vi "Facade.vi"(0 "Data In":T6, 2 "Display State In":T3, 3 "Container State":T5) -> (6 "Data Out":T6, 7 "Display State Out":T3, 8 "Action":T2)   [LabVIEW 2017, in "3D Comet.xctl"]
uses:
  <vilib>/Math Plots/3D Math Plots/3D Comet/3D Comet XCtrl/3D Comet.xctl
  <vilib>/Math Plots/3D Math Plots/3D Comet/3D Comet XCtrl/Data.ctl
  <vilib>/Math Plots/3D Math Plots/3D Plot/3D Plot Datatype/3D Plot Datatype.lvclass
  <vilib>/_xctls/Container State.ctl
  <vilib>/Math Plots/3D Math Plots/3D Comet/3D Comet XCtrl/State.ctl
  <vilib>/Math Plots/3D Math Plots/3D Comet/3D Comet/3D Comet.lvclass
  e:/builds/penguin/labview/branches/2017/dev/dist/vi.lib/Math Plots/3D Math Plots/3D Plot/3D Plot/3D Plot.lvclass
  <vilib>/Math Plots/3D Math Plots/3D Plot/Action String/3DMathPlot Ctrl Act Queue.ctl
  <vilib>/Math Plots/3D Math Plots/3D Plot/Action String/3DMathPlot Ctrl Act Cluster.ctl
  <vilib>/Math Plots/3D Math Plots/3D Plot/Action String/3DMathPlot State Class.ctl
  <vilib>/_xctls/Action.ctl
  <vilib>/Math Plots/3D Math Plots/3D Plot/3D Plot/Typedef/Plot Action.ctl
  <vilib>/Math Plots/3D Math Plots/3D Plot/Action String/3DMathPlot Action String.ctl
  <vilib>/_xctls/XControlSupport.lvlib
  <vilib>/Math Plots/3D Math Plots/3D Plot/3D Plot/3D Plot.lvclass
panel:
  out "Export Image":picture
  out "3D Picture Control":refnum<vi>(3d-picture)
  in  "XY Graph":cluster{dbl, dbl}[](graph)
  out "Render Window":refnum<vi>
  in  "Projection Palette":T1
  out "Intensity Graph":dbl[][](graph)
  in  "Color Ramp Palette":cluster{"Active Plot":i32} {"Active Plot" items=["Plot-1"]}
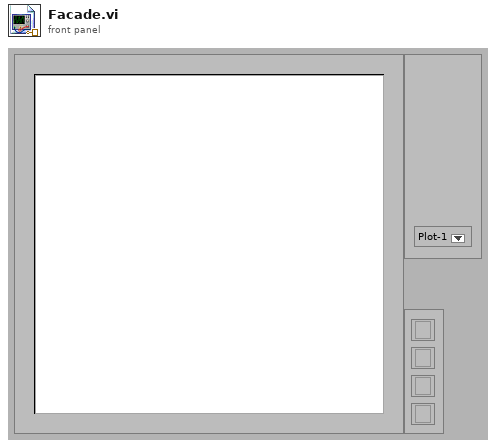
[diagram p1: front panel]
types:
  T1 = cluster{"XY Projection":bool, "XZ Projection":bool, "YZ Projection":bool, "3D Projection":bool}
  T2 = typedef "XControlSupport.lvlib/Action.ctl" = cluster{"Data Changed?":bool, "State Changed?":bool, "Action Name":string}
  T3 = typedef "3D Comet.xctl/State.ctl" = cluster{"3D Comet.lvclass":refnum<class "3D Comet.lvclass">, "Control Ref Queue":T4, "Main Frame Color":u32, "Ramp Palette Color":u32, "Projection Palette Color":u32}
  T4 = typedef "3DMathPlot Ctrl Act Queue.ctl" = refnum<queue>
  T5 = typedef "XControlSupport.lvlib/Container State.ctl" = cluster{"Indicator?":bool, "Run Mode?":bool, " Refnum":refnum<vi>}
  T6 = typedef "3D Comet.xctl/Data.ctl" = refnum<class "3D Plot Datatype.lvclass">[]
  T7 = typedef "3DMathPlot Ctrl Act Cluster.ctl" = cluster{"3D Picture Control":refnum<vi>, "Render Window Refnum":refnum<vi>, "XY Graph":refnum<vi>, "Intensity Graph":refnum<vi>, "Color Legend Palette":refnum<vi>, "Projection Palette":refnum<vi>, "XControl  Ref":refnum<vi>, "Facade Ref":refnum<vi>, "Export Image Ref":refnum<vi>, "Clear Data Flag":bool, "Display State Change Class":T8}
  T8 = typedef "3DMathPlot State Class.ctl" = enum16{"Update All Objects (Undo)", "Update Light Object Only", "Update Axis Object Only", "Update Plot Object Only", "Update Cursor Object Only", "Update Axis Plot Cursor Objects", "No Update"}
  T9 = typedef "3D Plot.lvclass/Plot Action.ctl" = cluster{"Light Action":enum16{"Update", "Remove", "Nothing"}, "Axis Action":enum16{"Update", "Remove", "Nothing"}, "Plot Action":enum16{"Update", "Remove", "Nothing"}, "Cursor Action":enum16{"Update", "Remove", "Nothing"}, "Fast Draw Action":enum16{"Update", "Remove", "Nothing"}}
  T10 = enum32{"Towards X-Y Plane", "Towards X-Z Plane", "Towards Y-Z Plane", "User Defined"}
  T11 = typedef "3D Plot.lvclass/Actual Transform.ctl" = cluster{"Scale Cluster":cluster{"X Scale":sgl, "Y Scale":sgl, "Z Scale":sgl}, "Translate Cluster":cluster{"X Translate":sgl, "Y Translate":sgl, "Z Translate":sgl}, "Actual Range":T12}
  T12 = typedef "3D Plot.lvclass/Range Clusters.ctl" = cluster{"X Range":cluster{"Max X":sgl, "Min X":sgl}, "Y Range":cluster{"Max Y":sgl, "Min Y":sgl}, "Z Range":cluster{"Max Z":sgl, "Min Z":sgl}}
  T13 = typedef "3D Plot.lvclass/Multiplot Representation.ctl" = cluster{"Plot Represention Array":T14[], "Max Range":T12}
  T14 = typedef "3D Plot.lvclass/Plot Representation.ctl" = cluster{"Plot ID":i32, "Plot Range":T12, "Mesh Data":T15, "Dimension":cluster{"X Dimension":i32, "Y Dimension":i32}, "Ramp Range":T12}
  T15 = typedef "3D Plot.lvclass/Mesh Data.ctl" = cluster{"Index Array":u32[], "Vertex Array":cluster{"X":sgl, "Y":sgl, "Z":sgl}[], "Normal Array":cluster{"X":sgl, "Y":sgl, "Z":sgl}[], "Color Index Array":i32[]}
  T16 = typedef "3D Plot.lvclass/Object Cluster.ctl" = cluster{"Root Scene Object":refnum<vi>, "Fast Root Scene Object":refnum<vi>}
  T17 = typedef "3DMathPlot Action String.ctl" = u16
  T18 = typedef "3D Plot.lvclass/Property Cluster.ctl" = cluster{"Graph Property":T19, "Light Property":T23, "Axis Property":T25, "Value Pair Property":T31, "Format Property":T33, "Cursor Property Array":T34, "Appearance Property":T43}
  T19 = typedef "3D Plot.lvclass/Graph Property.ctl" = cluster{"General Property":T20, "View Property":T21, "Grid Plane":T22}
  T20 = typedef "3D Plot.lvclass/General Property.ctl" = cluster{"Plot Area Color":u32, "Fast Draw?":bool, "Clip Data?":bool}
  T21 = typedef "3D Plot.lvclass/View Property.ctl" = cluster{"Projection Mode":enum16{"Orthographic", "Perspective"}, "View Direction":enum32{"Towards X-Y Plane", "Towards X-Z Plane", "Towards Y-Z Plane", "User Defined"}, "User Defined View Direction":cluster{"View Latitude":sgl, "View Longitude":sgl, "View Distance":sgl}}
  T22 = typedef "3D Plot.lvclass/Grid Plane.ctl" = cluster{"Grid Plane Visible":cluster{"Draw Grid Plane X-Y":bool, "Draw Grid Plane Y-Z":bool, "Draw Grid Plane X-Z":bool}, "Grid Antialiasing":bool, "Grid Frame Color":u32}
  T23 = typedef "3D Plot.lvclass/Light Property.ctl" = cluster{"Enable Lighting?":bool, "Ambient Color":u32, "Light Array":T24[]}
  T24 = typedef "3D Plot.lvclass/Light Specific.ctl" = cluster{"Enable Light?":bool, "Light Color":u32, "Light Latitude":sgl, "Light Longitude":sgl, "Light Distance":sgl, "Attenuation":enum16{"None", "Linear", "Quadratic"}}
  T25 = typedef "3D Plot.lvclass/Axis Property.ctl" = cluster{"Caption Property":T26, "Label Property":T27, "Range Property":T28, "Grid Property":T29, "Ticks Property":T30}
  T26 = typedef "3D Plot.lvclass/Caption Property.ctl" = cluster{"Show Caption":cluster{"Show Normal X Caption":bool, "Show Normal Y Caption":bool, "Show Normal Z Caption":bool, "Show Opposite X Caption":bool, "Show Opposite Y Caption":bool, "Show Opposite Z Caption":bool}, "Caption Color":cluster{"Caption Color X":u32, "Caption Color Y":u32, "Caption Color Z":u32}, "Caption Size":cluster{"Caption Size X":u16, "Caption Size Y":u16, "Caption Size Z":u16}, "Caption String":cluster{"Caption X":string, "Caption Y":string, "Caption Z ":string}}
  T27 = typedef "3D Plot.lvclass/Label Property.ctl" = cluster{"Show Label":cluster{"Show Normal X Label":bool, "Show Normal Y Label":bool, "Show Normal Z Label":bool, "Show Opposite X Label":bool, "Show Opposite Y Label":bool, "Show Opposite Z Label":bool}, "Label Color":cluster{"Label Color X":u32, "Label Color Y":u32, "Label Color Z":u32}, "Label Size":cluster{"Label Size X":u16, "Label Size Y":u16, "Labe Size Z":u16}}
  T28 = typedef "3D Plot.lvclass/Range Property.ctl" = cluster{"Range Cluster":T12, "Auto Range":cluster{"Auto Range X":bool, "Auto Range Y":bool, "Auto Range Z":bool}, "Inverted":cluster{"Inverted X":bool, "Inverted Y":bool, "Inverted Z":bool}, "Logarithm":cluster{"Logarithm X":bool, "Logarithm Y":bool, "Logarithm Z":bool}}
  T29 = typedef "3D Plot.lvclass/Grid Property.ctl" = cluster{"Major Grid Visible":cluster{"Draw Major Grid X":bool, "Draw Major Grid Y":bool, "Draw Major Grid Z":bool}, "Major Grid Color":cluster{"Major Grid Color X":u32, "Major Grid Color Y":u32, "Major Grid Color Z":u32}, "Minor Grid Visible":cluster{"Draw Minor Grid X":bool, "Draw Minor Grid Y":bool, "Draw Minor Grid Z":bool}, "Minor Grid Color":cluster{"Minor Grid Color X":u32, "Minor Grid Color Y":u32, "Minor Grid Color Z":u32}}
  T30 = typedef "3D Plot.lvclass/Tick Property.ctl" = cluster{"Major Tick Visible":cluster{"Draw Major Tick X":bool, "Draw Major Tick Y":bool, "Draw Major Tick Z":bool}, "Major Tick Color":cluster{"Major Tick Color X":u32, "Major Tick Color Y":u32, "Major Tick Color Z":u32}, "Major Count":cluster{"Major Count X":u16, "Major Count Y":u16, "Major Count Z":u16}, "Minor Tick Visible":cluster{"Draw Minor Tick X":bool, "Draw Minor Tick Y":bool, "Draw Minor Tick Z":bool}, "Minor Tick Color":cluster{"Minor Tick Color X":u32, "Minor Tick Color Y":u32, "Minor Tick Color Z":u32}, "Minor Count":cluster{"Minor Count X":u16, "Minor Count Y":u16, "Minor Count Z":u16}}
  T31 = typedef "3D Plot.lvclass/Value Pair Property.ctl" = T32[]
  T32 = typedef "3D Plot.lvclass/Value Pair Cluster.ctl" = cluster{"Value Pair Array":cluster{"Value":sgl, "Name":string}[], "Show Tick":bool, "Show Grid":bool, " Label Mode":enum16{"Name", "Value", "None"}}
  T33 = typedef "3D Plot.lvclass/Format Property.ctl" = string[]
  T34 = typedef "3D Plot.lvclass/Cursor Property Array.ctl" = T35[]
  T35 = typedef "3D Plot.lvclass/Cursor Property.ctl" = cluster{"Cursor Visible":bool, "Cursor Enable":bool, "Cursor Position":T36, "Cursor Point":T37, "Cursor Line":T39, "Cursor Plane":T41, "Cursor Text":T42}
  T36 = typedef "3D Plot.lvclass/Cursor Position.ctl" = cluster{"Cursor Plot ID":i32, "Cursor X":sgl, "Cursor Y":sgl, "Cursor Z":sgl, "Cursor Snap To":enum16{"Fixed", "Nearest Plot", "Snap to Plot"}}
  T37 = typedef "3D Plot.lvclass/Cursor Point.ctl" = cluster{"Cursor Point Color":u32, "Cursor Point Size":sgl, "Cursor Point Style":T38}
  T38 = typedef "3D Plot.lvclass/Sprite Type.ctl" = enum16{"None", "Empty Square", "Solid Square", "Empty Diamond", "Solid Diamond", "Empty Circle", "Solid Circle", "Asterisk", "Bold X", "Wireframe Sphere", "Solid Sphere", "Wireframe Cube", "Solid Cube"}
  T39 = typedef "3D Plot.lvclass/Cursor Line.ctl" = cluster{"Cursor Line Color":u32, "Cursor Line Width":sgl, "Cursor Line Style":T40}
  T40 = typedef "3D Plot.lvclass/Line Type.ctl" = enum16{"None", "Solid", "Dash", "Dot", "Dash Dot"}
  T41 = typedef "3D Plot.lvclass/Cursor Plane.ctl" = cluster{"Cursor Plane Color":u32, "Cursor Plane Opacity":sgl, "Draw Cursor Plane X-Z":bool, "Draw Cursor Plane Y-Z":bool, "Draw Cursor Plane X-Y":bool}
  T42 = typedef "3D Plot.lvclass/Cursor Text.ctl" = cluster{"Cursor Text":string, "Cursor Text Size":u16, "Cursor Show Position":bool, "Cursor Show Name":bool, "Cursor Text Color":u32, "Background Color":u32, "Background Opacity":sgl}
  T43 = typedef "3D Plot.lvclass/Apearance Property.ctl" = cluster{"Visibility":T44, "Active Index":cluster{"Active Plot":i32, "Active Cursor":i32, "Active Axis":enum16{"X-axis", "Y-axis", "Z-axis"}, "Active Value Pair":enum16{"X-axis", "Y-axis", "Z-axis"}, "Active Light":enum16{"Light 0", "Light 1", "Light 2", "Light 3"}}, "Backup Data":cluster{"Plot Name":string[]}}
  T44 = typedef "3D Plot.lvclass/Item Visibility.ctl" = cluster{"Projection Palette":bool, "Color Ramp Palette":bool}
  T45 = typedef "LVPoint32TypeDef.ctl" = cluster{"Horizontal":i32, "Vertical":i32}
  T46 = typedef "LVRangeTypeDef.ctl" = cluster{"Minimum":dbl, "Maximum":dbl, "Increment":dbl, "Minor Increment":dbl, "Start":dbl}
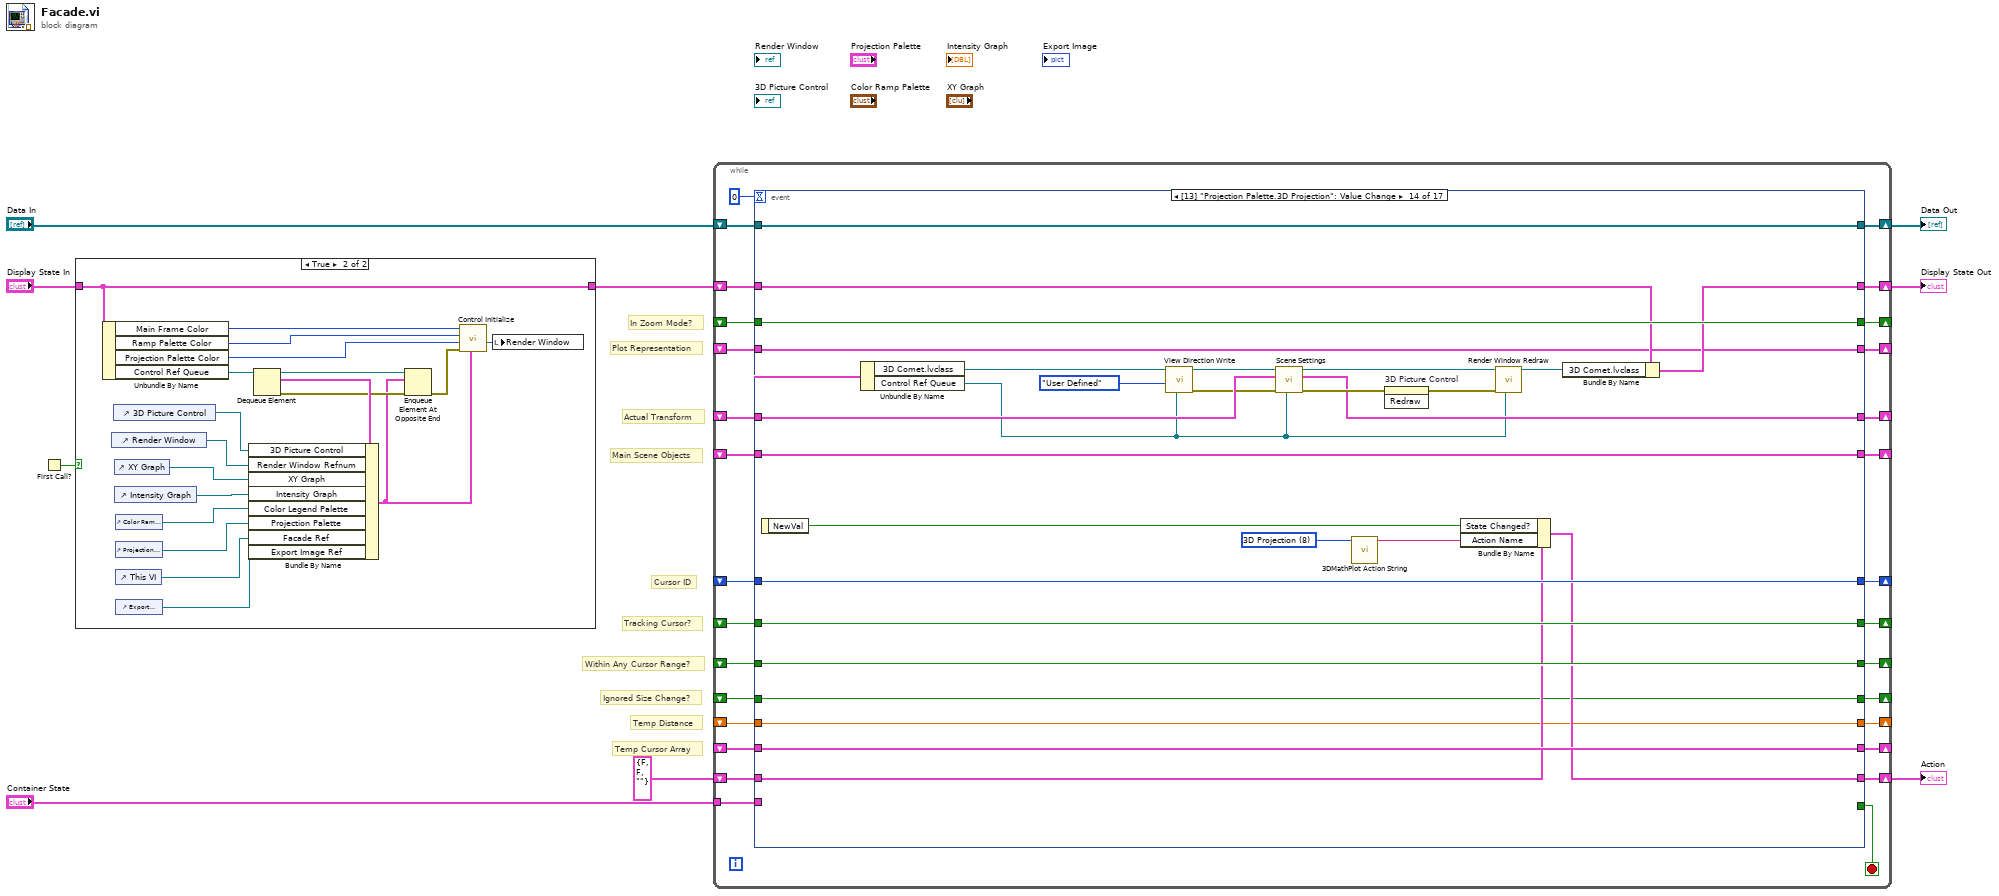
[diagram p0: block diagram]
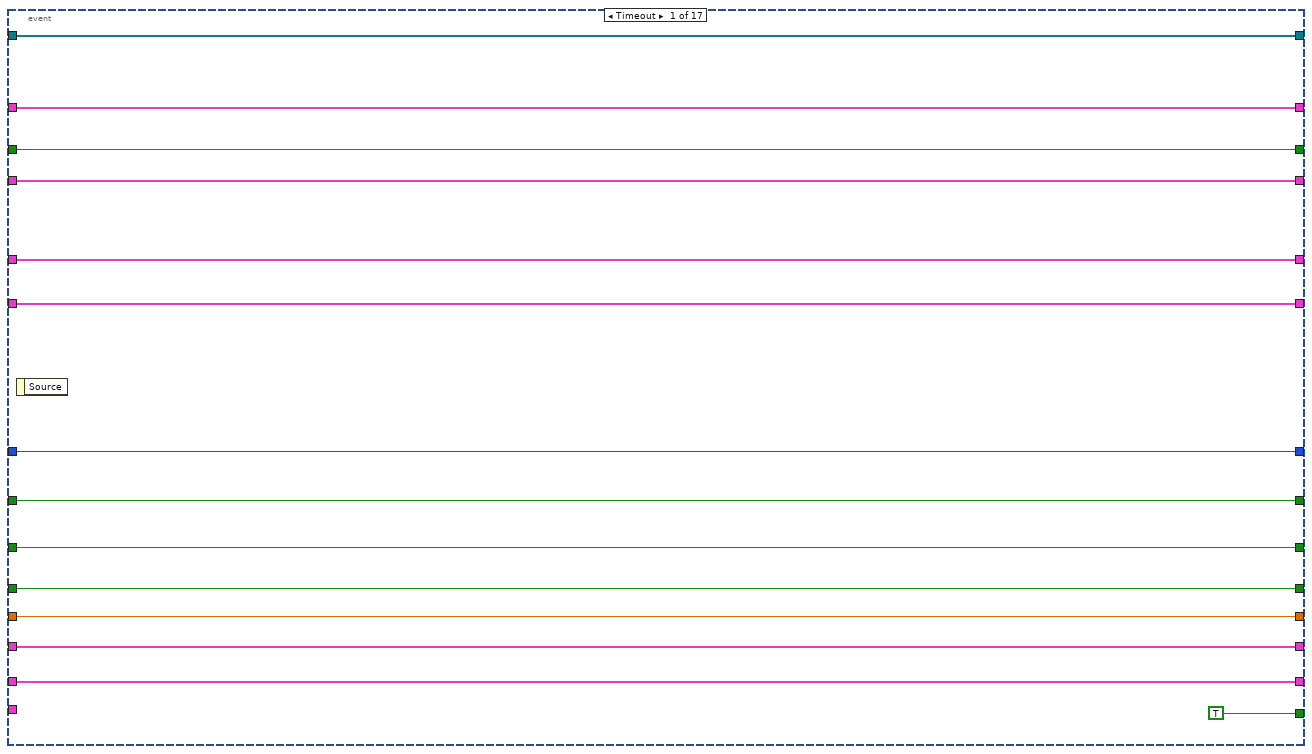
[diagram p3: hidden frame]
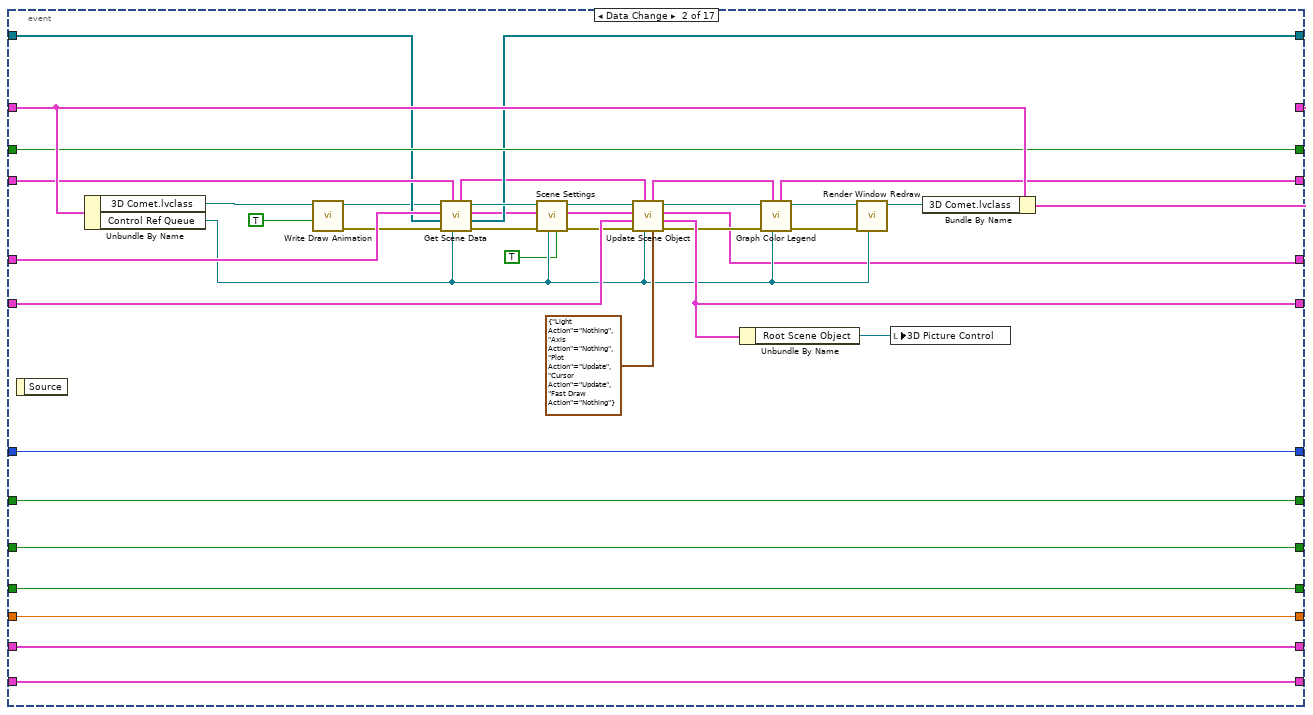
[diagram p4: hidden frame]
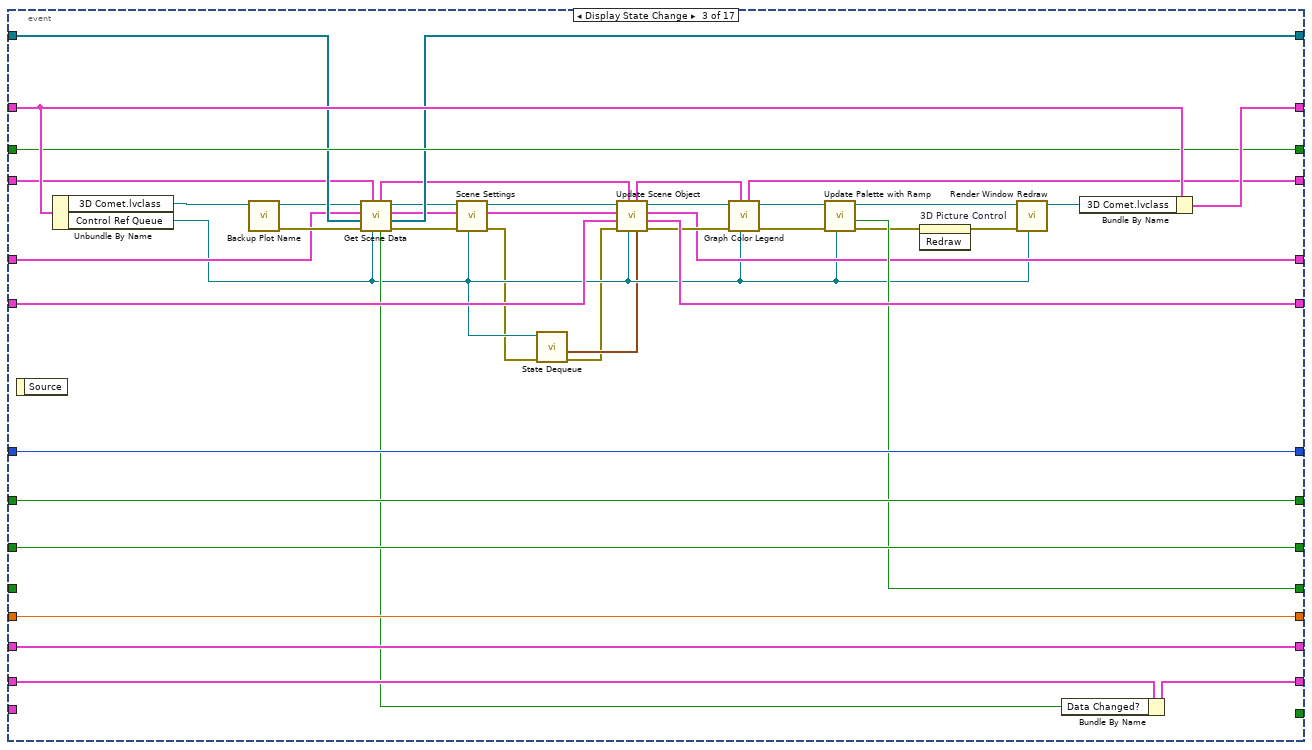
[diagram p5: hidden frame]
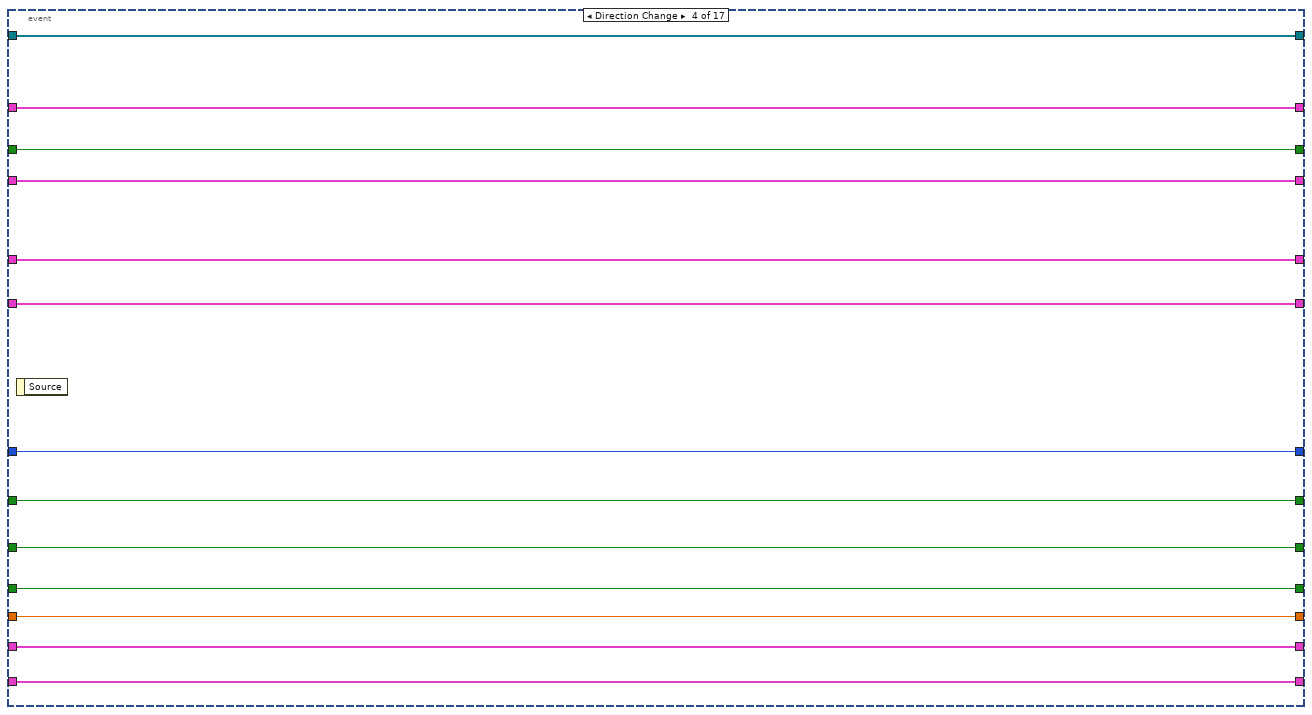
[diagram p6: hidden frame]
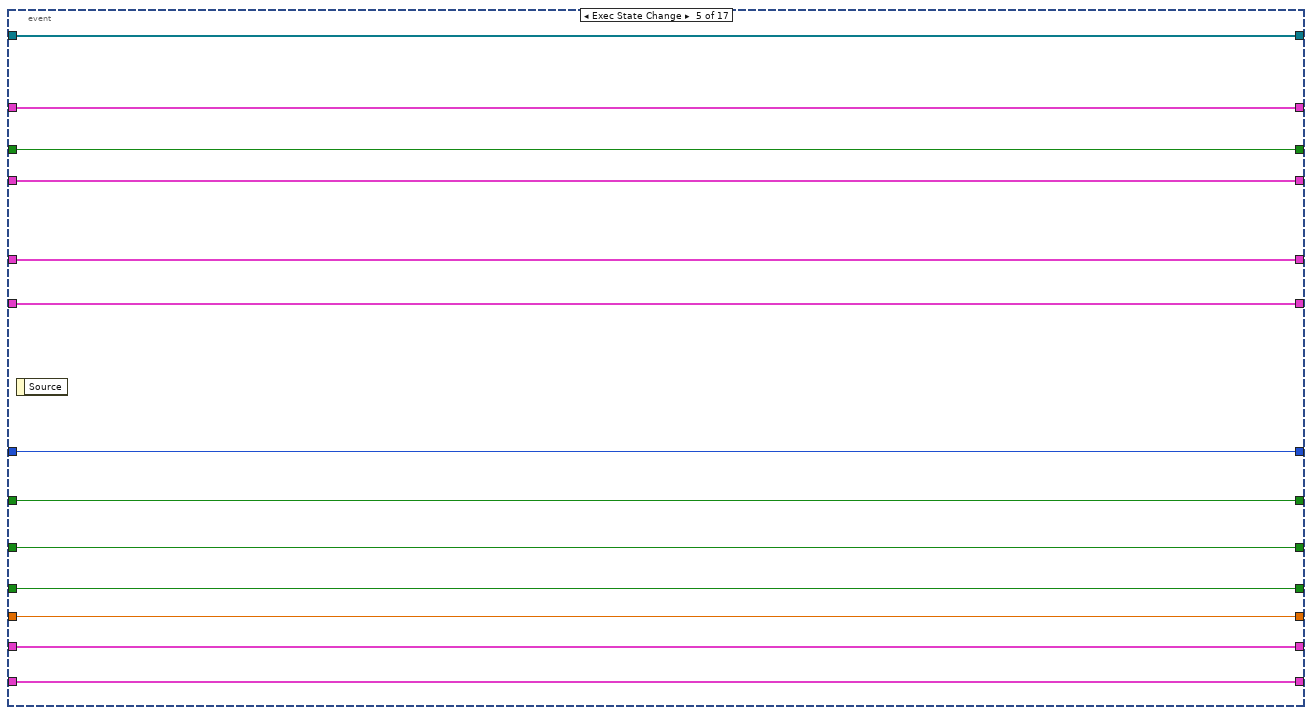
[diagram p7: hidden frame]
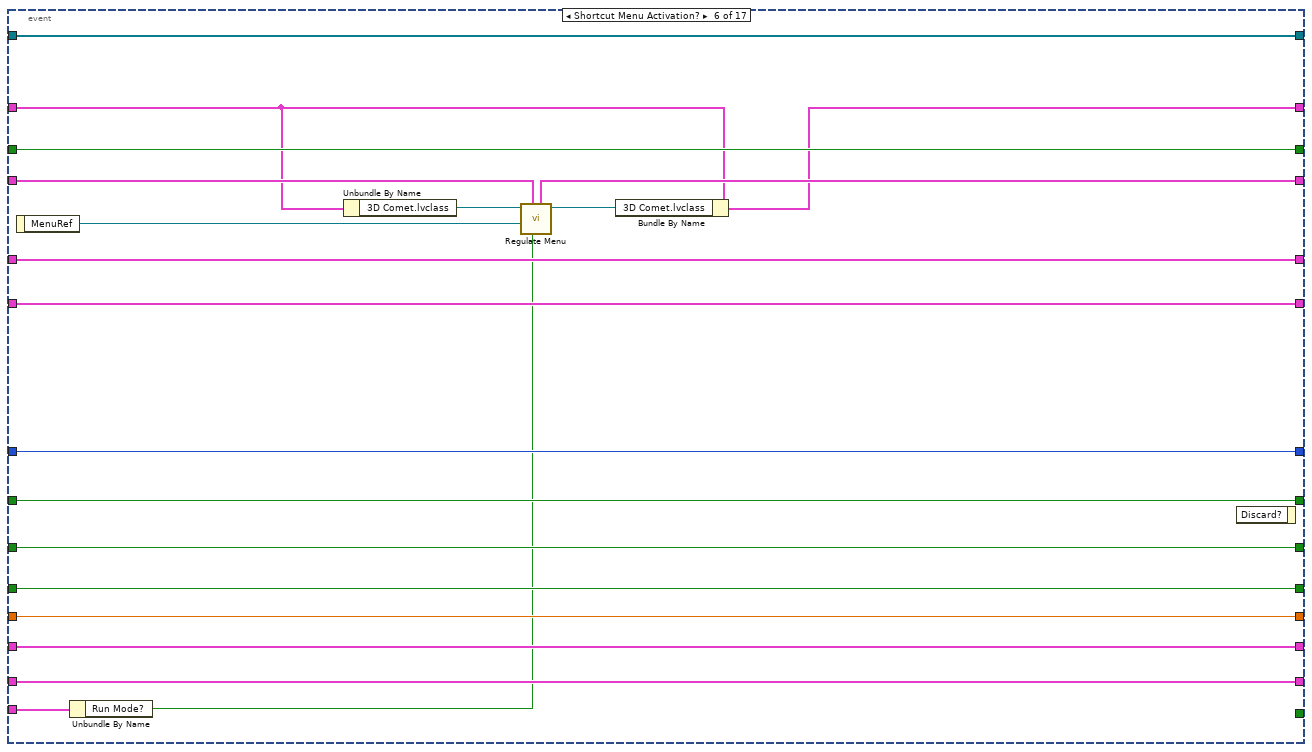
[diagram p8: hidden frame]
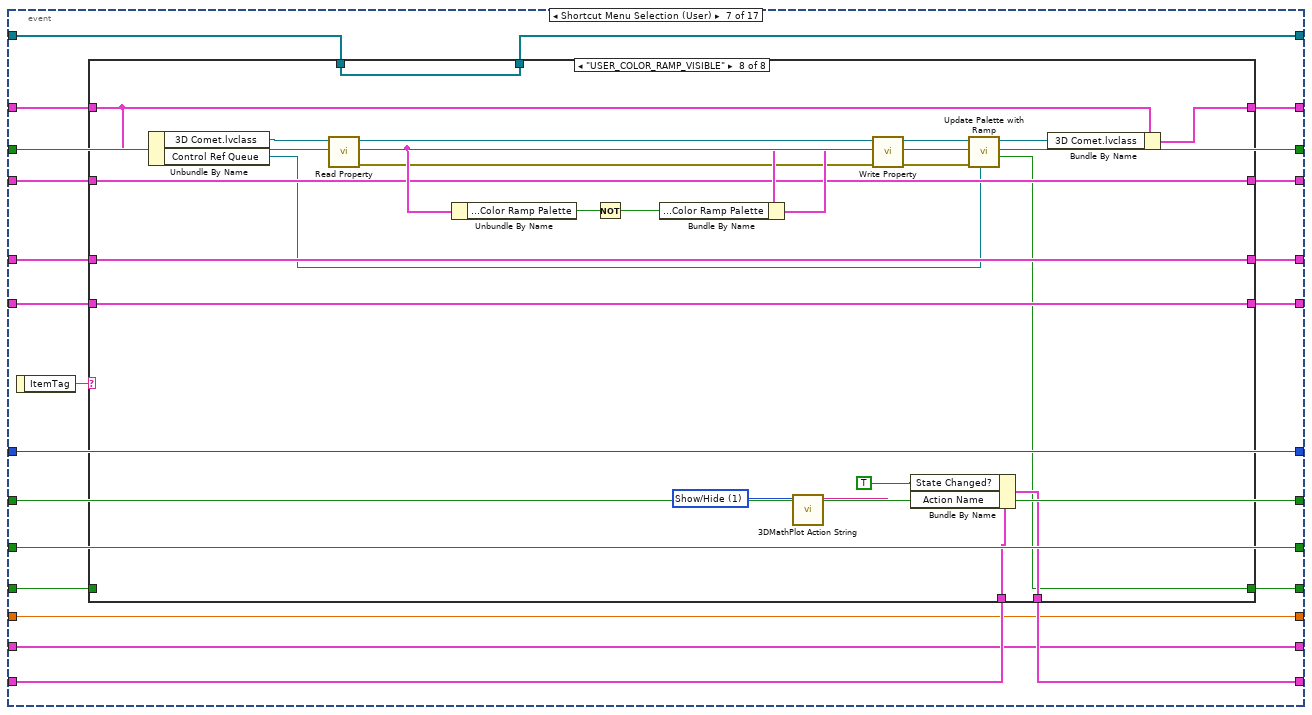
[diagram p9: hidden frame]
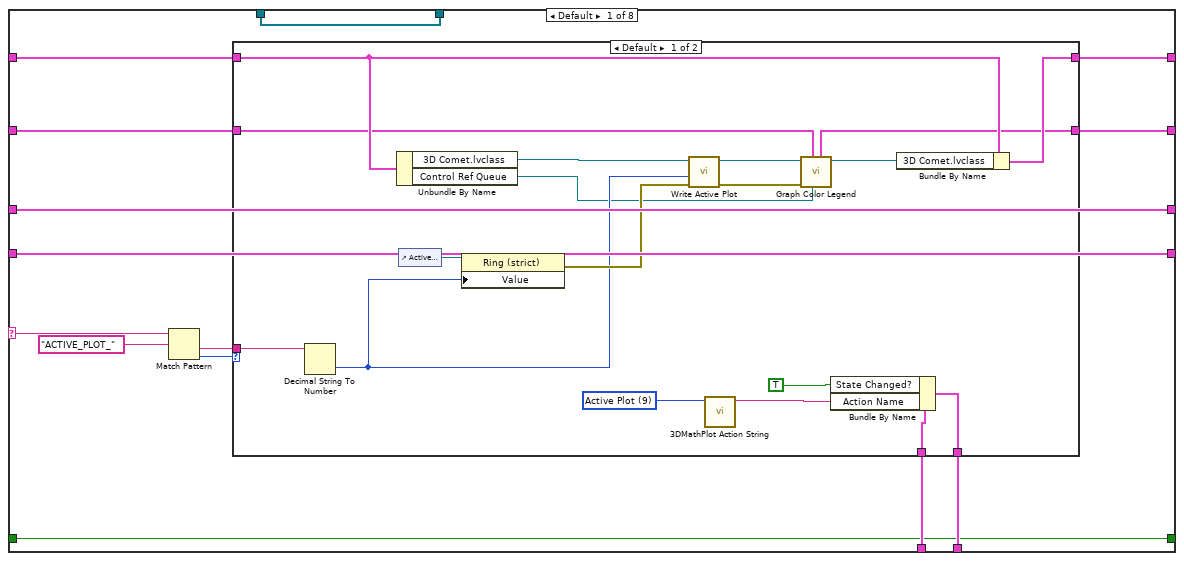
[diagram p10: hidden frame]
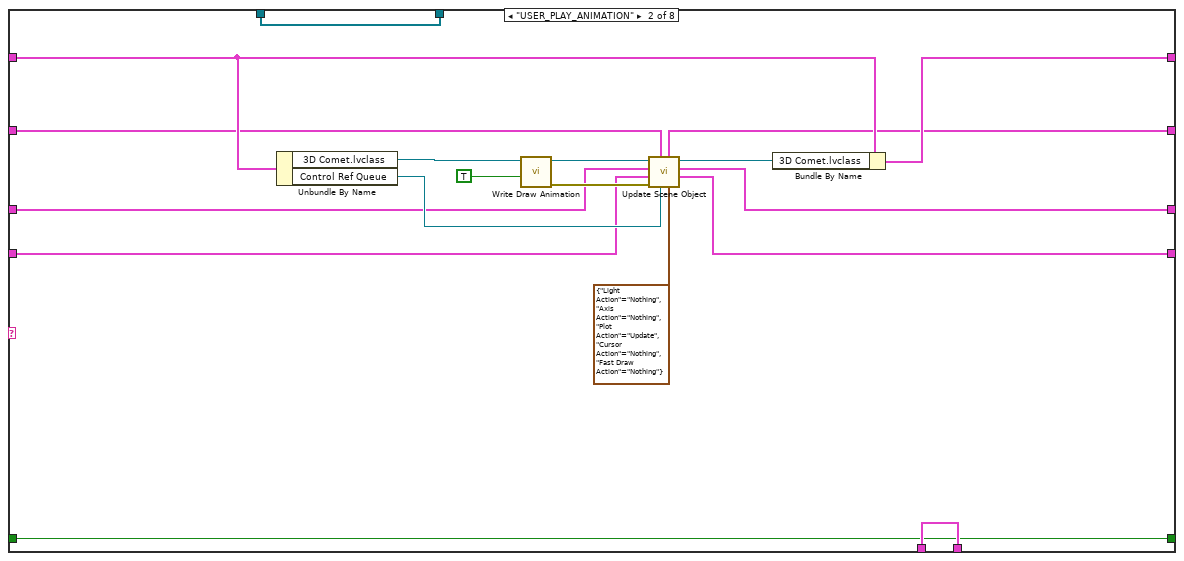
[diagram p12: hidden frame]
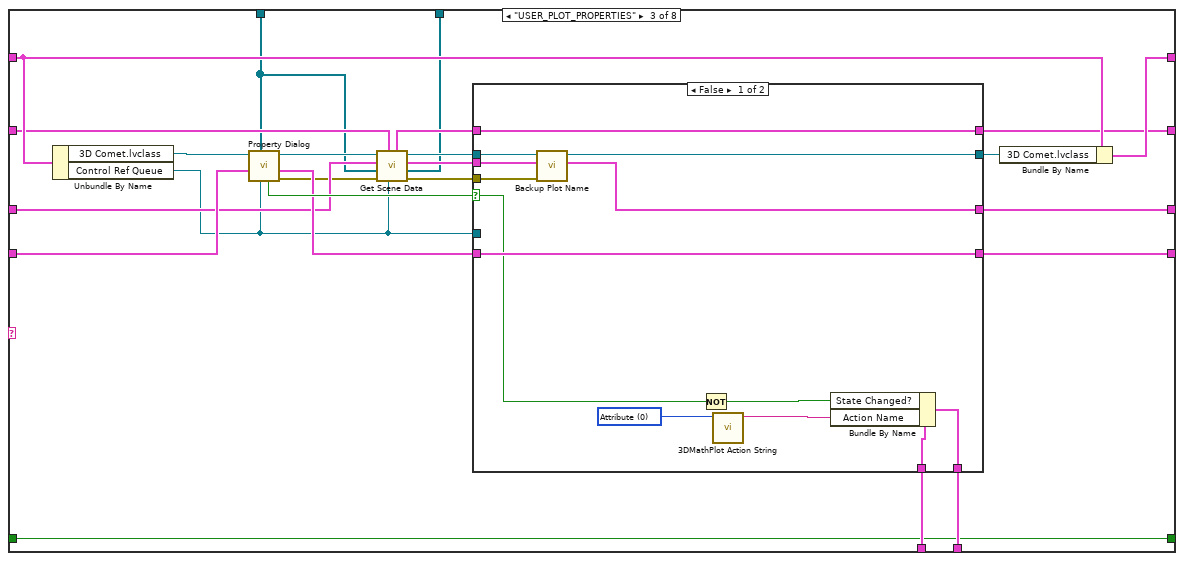
[diagram p13: hidden frame]
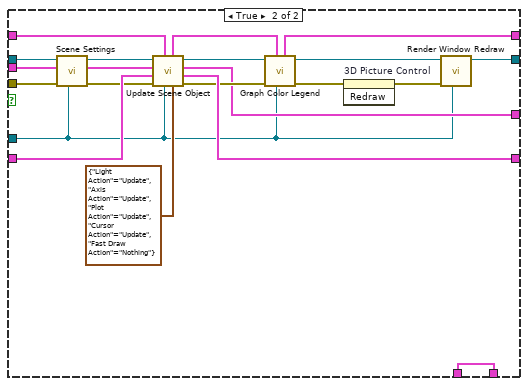
[diagram p14: hidden frame]
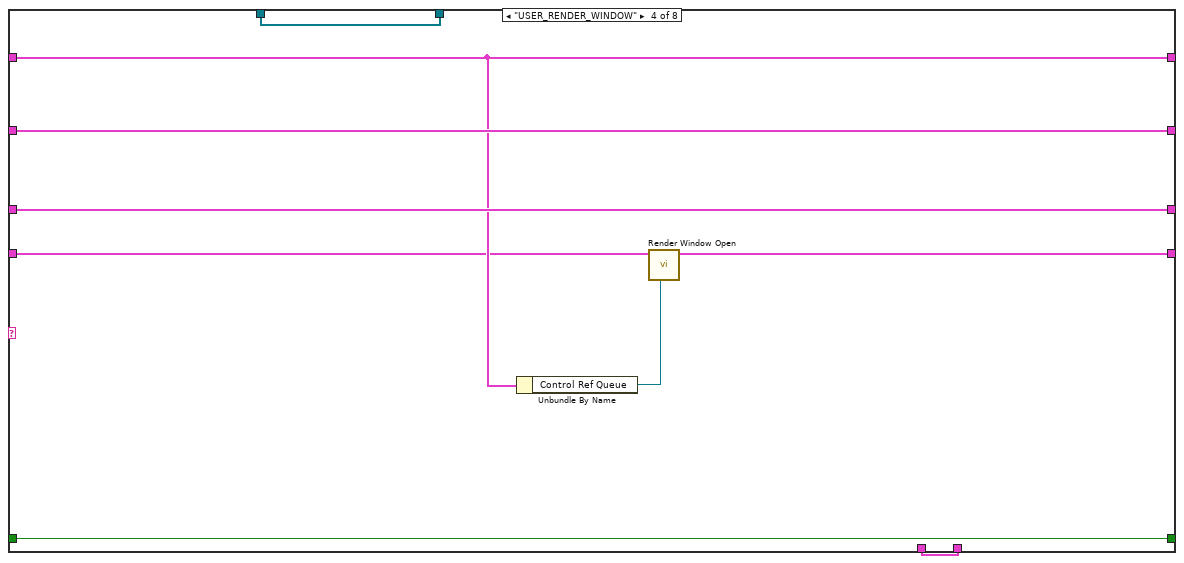
[diagram p15: hidden frame]
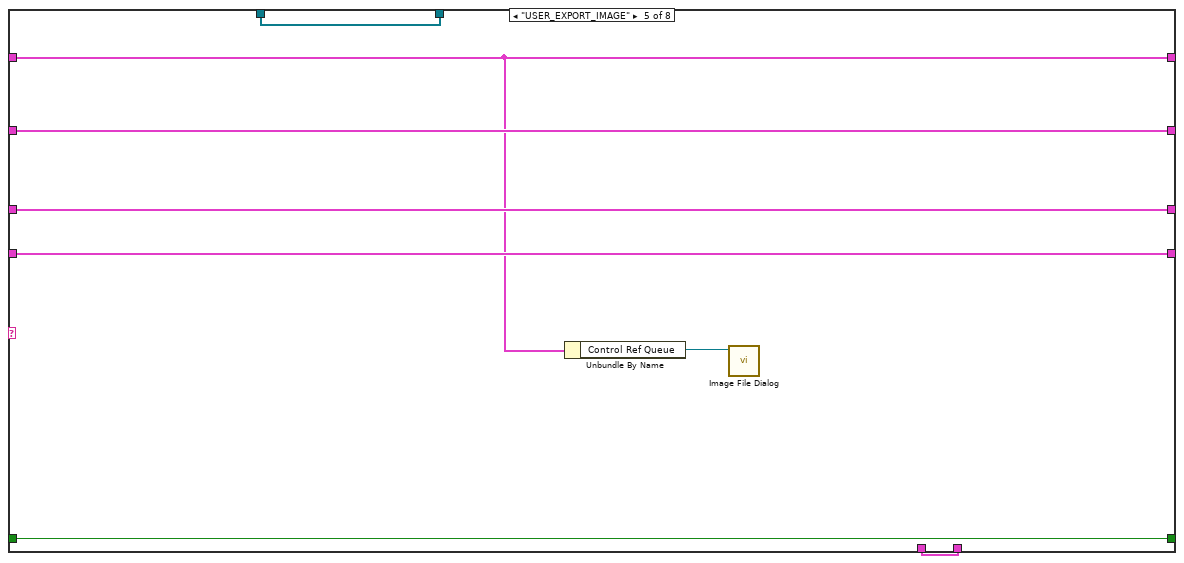
[diagram p16: hidden frame]
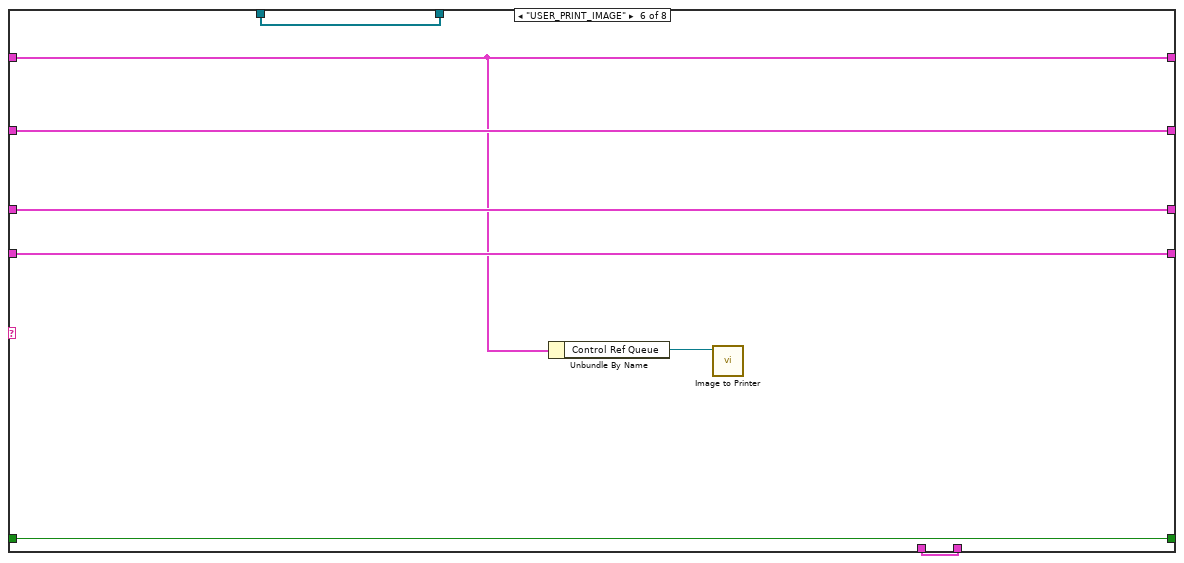
[diagram p17: hidden frame]
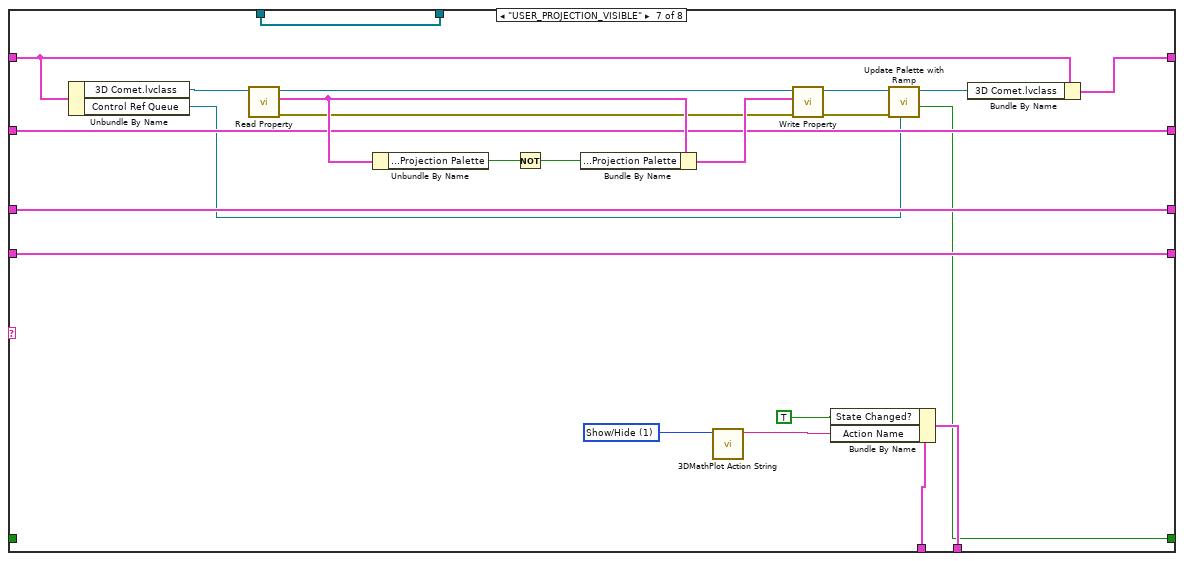
[diagram p18: hidden frame]
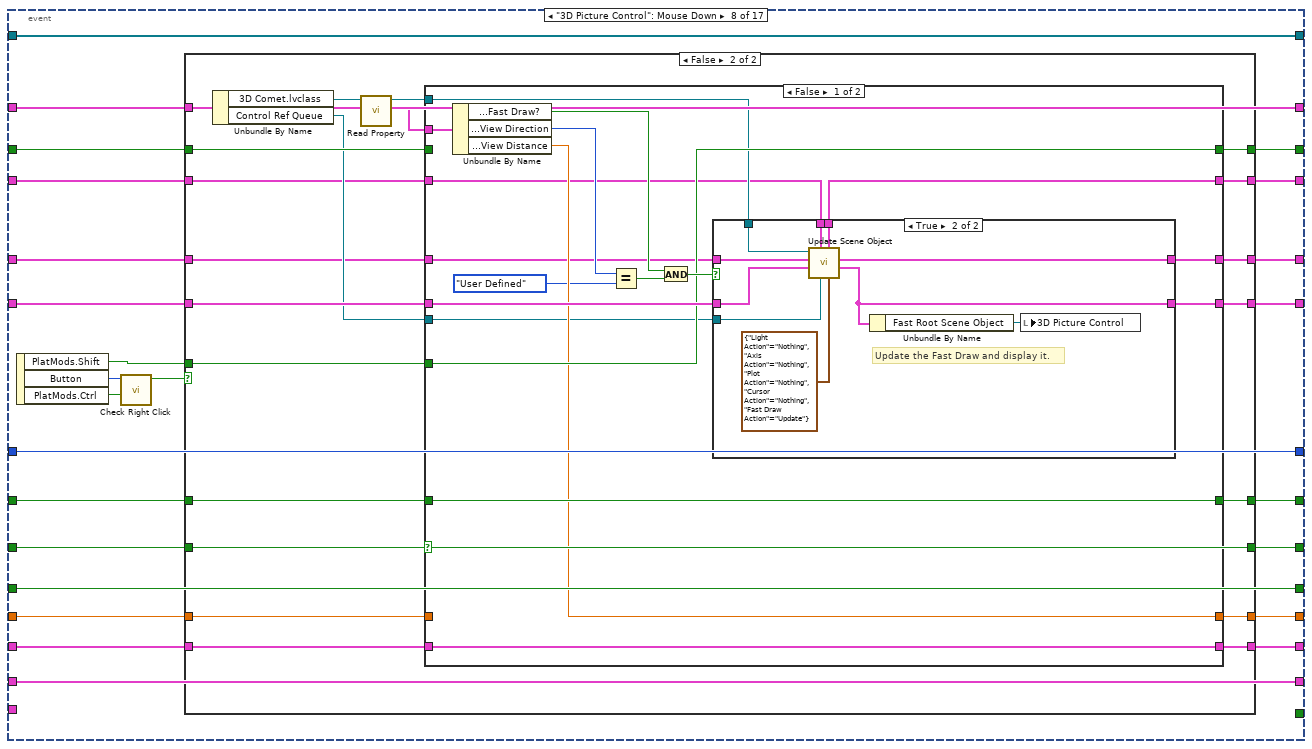
[diagram p19: hidden frame]
diagram:
  # "Ignored Size Change?"
  # "Actual Transform"
  # "Temp Cursor Array"
  # "Temp Distance"
  # "Within Any Cursor Range?"
  # "Tracking Cursor?"
  # "Cursor ID"
  # "Plot Representation"
  # "In Zoom Mode?"
  # "Main Scene Objects"
  n1 = First Call?() -> (First Call?: T/F=w4:bool)
  n2 = case shown="True" w4 {
    tunnel: [w10 w15] -> w3
    tunnel: "Display State In" -> [w10 w15]
    frame False {
    }
    frame True {
      n3 = Unbundle By Name(w15) -> ("Main Frame Color"=w13:u32, "Ramp Palette Color"=w12:u32, "Projection Palette Color"=w11:u32, "Control Ref Queue"=w16:T4)
      n4 = control-ref of="Render Window"() -> (w27:refnum<vi>)
      n5 = control-ref of="3D Picture Control"() -> (w28:refnum<vi>)
      n6 = control-ref of="XY Graph"() -> (w22:refnum<vi>)
      n7 = control-ref of="Intensity Graph"() -> (w26:refnum<vi>)
      n8 = control-ref of="Color Ramp Palette"() -> (w25:refnum<vi>)
      n9 = control-ref of="Projection Palette"() -> (w24:refnum<vi>)
      n10 = control-ref of="This VI"() -> (w23:refnum<vi>)
      n11 = control-ref of="Export Image"() -> (w14:refnum<vi>)
      n12 = Dequeue Element(queue=w16) -> (queue out=w20:T4, element=w21:T7, error out=w19:errorcluster)  [unwired: 1 in, 2 out]
      n13 = Bundle By Name(cluster=w21, "3D Picture Control"=w28, "Render Window Refnum"=w27, "XY Graph"=w22, "Intensity Graph"=w26, "Color Legend Palette"=w25, "Projection Palette"=w24, "Facade Ref"=w23, "Export Image Ref"=w14) -> (w17:T7)
      n14 = Enqueue Element At Opposite End(queue=w20, element=w17, error in (no error)=w19) -> (error out=w18:errorcluster)  [unwired: 3 out]
      n15 = call <vilib>:"Control Initialize.vi"("Control Ref Cluster"=w17, "error in (no error)"=w18, "Projection Palette Color"=w11, "Ramp Palette Color"=w12, "Main Frame Color"=w13) -> ("New Window Refnum"=w29:refnum<vi>)  [unwired: 6 out]
      n16 = local write "Render Window"(w29) -> ()
    }
  }
  n17 = while {
    shift-right: [w57] -> w7
    shift-left: w3 -> [w58]
    tunnel: "Container State" -> [w54]
    shift-right: [w53] -> w9
    shift-left: "Data In" -> [w48]
    shift-right: [w51] -> w6
    shift-left: T2 {"Data Changed?"=FALSE, "State Changed?"=FALSE, "Action Name"=""} ("Action") -> [w52]
    shift-right: [w50] -> _
    shift-left: _ -> [w49]
    shift-right: [w47] -> _
    shift-left: _ -> [w34]
    shift-right: [w45] -> _
    shift-left: _ -> [w46]
    shift-right: [w44] -> _
    shift-left: _ -> [w43]
    shift-right: [w41] -> _
    shift-left: _ -> [w42]
    shift-right: [w40] -> _
    shift-left: _ -> [w39]
    shift-right: [w38] -> _
    shift-left: _ -> [w37]
    shift-right: [w36] -> _
    shift-left: _ -> [w35]
    shift-right: [w33] -> _
    shift-left: _ -> [w32]
    shift-right: [w31] -> _
    shift-left: _ -> [w30]
    stop <- w56 stop-if-true
    n18 = event shown="[13] \"Projection Palette.3D Projection\": Value Change" {
      selector: _ -> [_ _ _ _ _ _ _ _ _ _ _ _ _ _ _ _ _]
      dyn-events: _ -> [_ _ _ _ _ _ _ _ _ _ _ _ _ _ _ _ _]
      timeout: 0 -> [_ _ _ _ _ _ _ _ _ _ _ _ _ _ _ _ _]
      tunnel: w58 -> [w60 w110 w150 w164 w177 w181 w214 w419 w507 w590 w616 w643 w670 w697 w721 w752 w768]
      tunnel: [w60 w109 w149 w164 w177 w180 w213 w419 w504 w590 w613 w642 w669 w696 w720 w751 w767] -> w57
      tunnel: [TRUE _ _ _ _ _ _ _ _ _ _ _ _ _ _ _ _] -> w56
      tunnel: w54 -> [_ _ _ _ _ w187 _ _ _ _ _ _ _ _ _ _ _]
      tunnel: w48 -> [w70 w86 w140 w163 w176 w197 w202 w423 w510 w594 w622 w649 w676 w703 w728 w761 w776]
      tunnel: [w70 w85 w141 w163 w176 w197 w201 w423 w510 w594 w622 w649 w676 w703 w728 w761 w776] -> w53
      tunnel: [w71 w100 w129 w162 w175 w195 w215 w422 w505 w593 w614 w640 w667 w694 w714 w748 w774] -> w51
      tunnel: w52 -> [w71 w100 w151 w162 w175 w195 w216 w422 w506 w593 w615 w641 w668 w695 w715 w749 w774]
      tunnel: [w62 w99 w143 w161 w174 w196 w217 w405 w508 w587 w606 w634 w660 w688 w709 w747 w775] -> w50
      tunnel: w49 -> [w62 w102 w144 w161 w174 w196 w218 w415 w509 w588 w606 w634 w660 w688 w709 w746 w775]
      tunnel: [w69 w107 w142 w160 w173 w194 w207 w402 w498 w591 w617 w648 w675 w702 w727 w756 w771] -> w47
      tunnel: w34 -> [w69 w107 w142 w160 w173 w194 w207 w418 w502 w592 w617 w648 w675 w702 w727 w756 w771]
      tunnel: w46 -> [w68 w106 w148 w159 w172 w193 w208 w421 w499 w586 w618 w647 w674 w701 w726 w757 w772]
      tunnel: [w68 w106 w148 w159 w172 w193 w208 w421 w499 w585 w618 w647 w674 w701 w726 w757 w772] -> w45
      tunnel: w43 -> [w67 w105 w147 w158 w171 w192 w209 w413 w501 w582 w619 w646 w673 w700 w725 w758 w773]
      tunnel: [w67 w105 w147 w158 w171 w192 w209 w406 w498 w582 w619 w646 w673 w700 w725 w758 w773] -> w44
      tunnel: w42 -> [w66 w104 w146 w157 w170 w191 w210 w412 _ _ w620 w645 w672 w699 w724 w759 w769]
      tunnel: [w66 w104 w146 w157 w170 w191 w210 w407 w498 w581 w620 w645 w672 w699 w724 w759 w769] -> w41
      tunnel: [w65 w103 w145 w156 w169 w190 w211 w408 w500 w584 w621 w644 w671 w698 w723 w760 w770] -> w40
      tunnel: w39 -> [w65 w103 w145 w156 w169 w190 w211 w410 w500 _ w621 w644 w671 w698 w723 w760 w770]
      tunnel: [w63 w79 w116 w155 w168 w183 w205 w403 w496 w580 w598 w631 w658 w685 w704 w734 w763] -> w38
      tunnel: w37 -> [w63 w88 w122 w155 w168 w184 w206 w417 w497 w580 w598 w631 w658 w685 w705 w730 w763]
      tunnel: w35 -> [w64 w87 w123 w154 w167 w189 w204 w416 w495 w579 w600 w630 w657 w684 w710 w733 w764]
      tunnel: [w64 w78 w117 w154 w167 w189 w203 w404 w494 w579 w599 w629 w656 w683 w710 w735 w764] -> w36
      tunnel: [w61 w96 w136 w153 w166 w188 w200 w420 w493 w578 w610 w637 w664 w691 w712 w743 FALSE] -> w33
      tunnel: w32 -> [w61 w96 _ w153 w166 w188 w199 w420 w493 w578 w610 w637 w664 w691 w712 w743 w766]
      tunnel: [w59 w90 w130 w152 w165 w186 w198 w409 w492 w572 w608 w635 w662 w689 w708 w736 w762] -> w31
      tunnel: w30 -> [w59 w90 w130 w152 w165 w186 w198 w411 w492 _ w608 w635 w662 w689 w708 w736 w762]
      event Timeout {
        n19 = event-data() -> ()  [unwired: 2 out]
      }
      event Data Change {
        n20 = event-data() -> ()  [unwired: 2 out]
        n21 = Unbundle By Name(w110) -> ("3D Comet.lvclass"=w77:refnum<class "3D Comet.lvclass">, "Control Ref Queue"=w82:T4)
        n22 = call-dynamic "Write Draw Animation.vi"("Draw Animation?"=TRUE, "3D Comet.lvclass in"=w77) -> ("error out"=w75:errorcluster, "3D Comet.lvclass out"=w76:refnum<class "3D Comet.lvclass">)  [unwired: 1 in, 7 out]
        n23 = call <vilib>:"Get Scene Data.vi"("Control Ref Queue"=w82, "Multiplot Representation In"=w88, "error in (no error)"=w75, "Data In"=w86, "Actual Transform In"=w87, "3D Plot.lvclass in"=w76) -> ("error out"=w83:errorcluster, "Data Out"=w85:refnum<class "3D Plot Datatype.lvclass">[], "Actual Transform Out"=w84:T11, "3D Plot.lvclass out"=w89:refnum<class "3D Comet.lvclass">, "Multiplot Representation Out"=w81:T13)  [unwired: 1 out]
        n24 = call <vilib>:"Scene Settings.vi"("Data Change Event?"=TRUE, "Control Ref Queue"=w82, "error in (no error)"=w83, "Actual Transform In"=w84, "3D Plot.lvclass in"=w89) -> ("error out"=w91:errorcluster, "Actual Transform Out"=w101:T11, "3D Plot.lvclass out"=w92:refnum<class "3D Comet.lvclass">)  [unwired: 2 in, 2 out]
        n25 = call <vilib>:"Update Scene Object.vi"("Action"=T9 {"Light Action"=enum."Nothing", "Axis Action"=enum."Nothing", "Plot Action"=enum."Update", "Cursor Action"=enum."Update", "Fast Draw Action"=enum."Nothing"}, "Control Ref Queue"=w82, "Multiplot Representation In"=w81, "error in (no error)"=w91, "Object Cluster In"=w102, "Actual Transform In"=w101, "3D Plot.lvclass in"=w92) -> ("error out"=w97:errorcluster, "Object Cluster Out"=w99:T16, "Actual Transform Out"=w78:T11, "3D Plot.lvclass out"=w98:refnum<class "3D Comet.lvclass">, "Multiplot Representation Out"=w80:T13)
        n26 = Unbundle By Name(w99) -> ("Root Scene Object"=w108:refnum<vi>)
        n27 = call-dynamic "Graph Color Legend.vi"("Control Ref Queue"=w82, "Multiplot Representation In"=w80, "error in (no error)"=w97, "3D Plot.lvclass in"=w98) -> ("error out"=w93:errorcluster, "3D Plot.lvclass out"=w94:refnum<class "3D Comet.lvclass">, "Multiplot Representation Out"=w79:T13)  [unwired: 2 in, 3 out]
        n28 = call <vilib>:"Render Window Redraw.vi"("Control Ref Queue"=w82, "error in (no error)"=w93) -> ()  [unwired: 1 in, 9 out]
        n29 = local write "3D Picture Control"(w108) -> ()
        n30 = Bundle By Name(cluster=w110, "3D Comet.lvclass"=w94) -> (w109:T3)
      }
      event Display State Change {
        n31 = event-data() -> ()  [unwired: 2 out]
        n32 = Unbundle By Name(w150) -> ("3D Comet.lvclass"=w115:refnum<class "3D Comet.lvclass">, "Control Ref Queue"=w114:T4)
        n33 = call-dynamic "Backup Plot Name.vi"("3D Comet.lvclass in"=w115) -> ("error out"=w124:errorcluster, "3D Comet.lvclass out"=w127:refnum<class "3D Comet.lvclass">)  [unwired: 1 in, 8 out]
        n34 = call <vilib>:"Get Scene Data.vi"("Control Ref Queue"=w114, "Multiplot Representation In"=w122, "error in (no error)"=w124, "Data In"=w140, "Actual Transform In"=w123, "3D Plot.lvclass in"=w127) -> ("error out"=w126:errorcluster, "Data Out"=w141:refnum<class "3D Plot Datatype.lvclass">[], "Actual Transform Out"=w121:T11, "3D Plot.lvclass out"=w125:refnum<class "3D Comet.lvclass">, "Data Cleaned?"=w128:bool, "Multiplot Representation Out"=w119:T13)
        n35 = call <vilib>:"Scene Settings.vi"("Control Ref Queue"=w114, "error in (no error)"=w126, "Actual Transform In"=w121, "3D Plot.lvclass in"=w125) -> ("error out"=w112:errorcluster, "Actual Transform Out"=w120:T11, "3D Plot.lvclass out"=w131:refnum<class "3D Comet.lvclass">)  [unwired: 3 in, 2 out]
        n36 = call <vilib>:"State Dequeue.vi"("error in (no error)"=w112, "Control Ref Queue"=w114) -> ("error out"=w111:errorcluster, "Action"=w113:T9)  [unwired: 8 out]
        n37 = call <vilib>:"Update Scene Object.vi"("Action"=w113, "Control Ref Queue"=w114, "Multiplot Representation In"=w119, "error in (no error)"=w111, "Object Cluster In"=w144, "Actual Transform In"=w120, "3D Plot.lvclass in"=w131) -> ("error out"=w138:errorcluster, "Object Cluster Out"=w143:T16, "Actual Transform Out"=w117:T11, "3D Plot.lvclass out"=w139:refnum<class "3D Comet.lvclass">, "Multiplot Representation Out"=w118:T13)
        n38 = call-dynamic "Graph Color Legend.vi"("Control Ref Queue"=w114, "Multiplot Representation In"=w118, "error in (no error)"=w138, "3D Plot.lvclass in"=w139) -> ("error out"=w134:errorcluster, "3D Plot.lvclass out"=w135:refnum<class "3D Comet.lvclass">, "Multiplot Representation Out"=w116:T13)  [unwired: 2 in, 3 out]
        n39 = call <vilib>:"Update Palette with Ramp.vi"("Control Ref Queue"=w114, "error in (no error)"=w134, "3D Plot.lvclass in"=w135) -> ("error out"=w133:errorcluster, "Ignore the size change?"=w136:bool, "3D Plot.lvclass out"=w137:refnum<class "3D Comet.lvclass">)  [unwired: 6 out]
        n40 = invoke on="3D Picture Control" class="SceneGraphDisp (strict)" method="Redraw"(error in=w133) -> (error out=w132:errorcluster)  [unwired: 2 in, 2 out]
        n41 = call <vilib>:"Render Window Redraw.vi"("Control Ref Queue"=w114, "error in (no error)"=w132) -> ()  [unwired: 1 in, 9 out]
        n42 = Bundle By Name(cluster=w151, "Data Changed?"=w128) -> (w129:T2)
        n43 = Bundle By Name(cluster=w150, "3D Comet.lvclass"=w137) -> (w149:T3)
      }
      event Direction Change {
        n44 = event-data() -> ()  [unwired: 2 out]
      }
      event Exec State Change {
        n45 = event-data() -> ()  [unwired: 2 out]
      }
      event Shortcut Menu Activation? {
        n46 = event-data() -> ("MenuRef"=w179:refnum<k9>)  [unwired: 1 out]
        n47 = Unbundle By Name(w187) -> ("Run Mode?"=w178:bool)
        n48 = Unbundle By Name(w181) -> ("3D Comet.lvclass"=w185:refnum<class "3D Comet.lvclass">)
        n49 = call <vilib>:"Regulate Menu.vi"("Run Mode?"=w178, "Multiplot Representation In"=w184, "MenuRef"=w179, "3D Plot.lvclass in"=w185) -> ("3D Plot.lvclass out"=w182:refnum<class "3D Comet.lvclass">, "Multiplot Representation Out"=w183:T13)  [unwired: 3 in, 3 out]
        n50 = Bundle By Name(cluster=w181, "3D Comet.lvclass"=w182) -> (w180:T3)
        n51 = event-data() -> ()  [unwired: 1 in, 2 out]
      }
      event Shortcut Menu Selection (User) {
        n52 = event-data() -> ("ItemTag"=w212:string)  [unwired: 1 out]
        n53 = case shown="\"USER_COLOR_RAMP_VISIBLE\"" w212 {
          selector: w212 -> [w231 _ _ _ _ _ _ _]
          tunnel: w214 -> [w228 w265 w295 w331 w338 w345 w366 w392]
          tunnel: [w227 w264 w294 w331 w338 w345 w365 w391] -> w213
          tunnel: w218 -> [w232 w260 w285 w329 w344 w352 w371 w390]
          tunnel: [w232 w256 w292 w328 w344 w352 w371 w390] -> w217
          tunnel: w216 -> [w224 w255 w288 w334 w343 w347 w374 w387]
          tunnel: [w225 w255 w287 w334 w343 w347 w373 w386] -> w215
          tunnel: w206 -> [w221 w259 w280 w335 w342 w351 w364 w389]
          tunnel: [w220 w258 w291 w335 w342 w351 w364 w389] -> w205
          tunnel: w204 -> [w219 w261 w278 w332 w339 w350 w363 w388]
          tunnel: [w219 w257 w289 w332 w339 w350 w363 w388] -> w203
          tunnel: w202 -> [w223 w262 w276 w336 w341 w349 w360 w383]
          tunnel: [w223 w262 w275 w336 w341 w349 w360 w383] -> w201
          tunnel: [w222 w254 w286 w333 w340 w346 w354 w377] -> w200
          tunnel: w199 -> [w222 w254 w286 w333 w340 w346 _ _]
          frame Default {
            n54 = Match Pattern(string=w231, regular expression="ACTIVE_PLOT_") -> (after substring=w226:string, offset past match=w229:i32)  [unwired: 3 out]
            n55 = case shown="Default" w229 {
              tunnel: w228 -> [w243 w253]
              tunnel: [w242 w253] -> w227
              tunnel: w226 -> [w249 _]
              tunnel: [w244 w252] -> w225
              tunnel: w224 -> [w245 w252]
              tunnel: w221 -> [w234 w251]
              tunnel: [w233 w251] -> w220
              frame Default {
                w246 = T17 9 items=["Attribute", "Show/Hide", "Cursor Move", "Zoom", "Mouse Drag", "XY Projection", "YZ Projection", "XZ Projection", "3D Projection", "Active Plot", "Scale"] ("Global String")
                n56 = Decimal String To Number(string=w249) -> (number=w239:i32)  [unwired: 3 out]
                n57 = Unbundle By Name(w243) -> ("3D Comet.lvclass"=w250:refnum<class "3D Comet.lvclass">, "Control Ref Queue"=w237:T4)
                n58 = control-ref of="Active Plot"() -> (w241:refnum<vi>)
                n59 = property class="Ring (strict)"(reference=w241, "Value"=w239) -> (error out=w240:errorcluster)  [unwired: 1 in, 1 out]
                n60 = call-dynamic "Write Active Plot.vi"("error in (no error)"=w240, "Active Plot"=w239, "3D Comet.lvclass in"=w250) -> ("error out"=w235:errorcluster, "3D Comet.lvclass out"=w236:refnum<class "3D Comet.lvclass">)  [unwired: 7 in]
                n61 = call <vilib>:"3DMathPlot Action String.vi"("Global String"=w246) -> ("String Out"=w247:string)  [unwired: 10 out]
                n62 = call-dynamic "Graph Color Legend.vi"("Control Ref Queue"=w237, "Multiplot Representation In"=w234, "error in (no error)"=w235, "3D Plot.lvclass in"=w236) -> ("3D Plot.lvclass out"=w238:refnum<class "3D Comet.lvclass">, "Multiplot Representation Out"=w233:T13)  [unwired: 2 in, 4 out]
                n63 = Bundle By Name(cluster=w245, "State Changed?"=TRUE ("Data Changed?"), "Action Name"=w247) -> (w244:T2)
                n64 = Bundle By Name(cluster=w243, "3D Comet.lvclass"=w238) -> (w242:T3)
              }
              frame -1 {
              }
            }
          }
          frame "USER_PLAY_ANIMATION" {
            n65 = Unbundle By Name(w265) -> ("3D Comet.lvclass"=w268:refnum<class "3D Comet.lvclass">, "Control Ref Queue"=w267:T4)
            n66 = call-dynamic "Write Draw Animation.vi"("Draw Animation?"=TRUE, "3D Comet.lvclass in"=w268) -> ("error out"=w263:errorcluster, "3D Comet.lvclass out"=w269:refnum<class "3D Comet.lvclass">)  [unwired: 1 in, 7 out]
            n67 = call <vilib>:"Update Scene Object.vi"("Action"=T9 {"Light Action"=enum."Nothing", "Axis Action"=enum."Nothing", "Plot Action"=enum."Update", "Cursor Action"=enum."Nothing", "Fast Draw Action"=enum."Nothing"}, "Control Ref Queue"=w267, "Multiplot Representation In"=w259, "error in (no error)"=w263, "Object Cluster In"=w260, "Actual Transform In"=w261, "3D Plot.lvclass in"=w269) -> ("Object Cluster Out"=w256:T16, "Actual Transform Out"=w257:T11, "3D Plot.lvclass out"=w266:refnum<class "3D Comet.lvclass">, "Multiplot Representation Out"=w258:T13)  [unwired: 1 out]
            n68 = Bundle By Name(cluster=w265, "3D Comet.lvclass"=w266) -> (w264:T3)
          }
          frame "USER_PLOT_PROPERTIES" {
            n69 = Unbundle By Name(w295) -> ("3D Comet.lvclass"=w293:refnum<class "3D Comet.lvclass">, "Control Ref Queue"=w272:T4)
            n70 = call-dynamic "Property Dialog.vi"("Control Ref Queue"=w272, "Data"=w276, "Object Cluster In"=w285, "3D Comet in"=w293) -> ("error out"=w274:errorcluster, "Object Cluster Out"=w283:T16, "3D Comet out"=w282:refnum<class "3D Comet.lvclass">, "Cancel?"=w284:bool)  [unwired: 1 in, 3 out]
            n71 = call <vilib>:"Get Scene Data.vi"("Control Ref Queue"=w272, "Multiplot Representation In"=w280, "error in (no error)"=w274, "Data In"=w276, "Actual Transform In"=w278, "3D Plot.lvclass in"=w282) -> ("error out"=w273:errorcluster, "Data Out"=w275:refnum<class "3D Plot Datatype.lvclass">[], "Actual Transform Out"=w277:T11, "3D Plot.lvclass out"=w281:refnum<class "3D Comet.lvclass">, "Multiplot Representation Out"=w279:T13)  [unwired: 1 out]
            n72 = case shown="False" w284 {
              selector: w284 -> [w297 _]
              tunnel: w283 -> [w305 w320]
              tunnel: w279 -> [w306 w311]
              tunnel: [w305 w327] -> w292
              tunnel: [w306 w314] -> w291
              tunnel: w281 -> [w300 w309]
              tunnel: w273 -> [w299 w310]
              tunnel: [w298 w324] -> w290
              tunnel: [w307 w313] -> w289
              tunnel: w277 -> [w307 w308]
              tunnel: w288 -> [w302 w321]
              tunnel: [w301 w321] -> w287
              tunnel: w272 -> [_ w312]
              frame False {
                w303 = T17 0 items=["Attribute", "Show/Hide", "Cursor Move", "Zoom", "Mouse Drag", "XY Projection", "YZ Projection", "XZ Projection", "3D Projection", "Active Plot", "Scale"] ("Global String")
                n73 = call-dynamic "Backup Plot Name.vi"("error in (no error)"=w299, "3D Comet.lvclass in"=w300) -> ("3D Comet.lvclass out"=w298:refnum<class "3D Comet.lvclass">)  [unwired: 9 out]
                n74 = Not(x=w297) -> (.not. x?=w296:bool)
                n75 = call <vilib>:"3DMathPlot Action String.vi"("Global String"=w303) -> ("String Out"=w304:string)  [unwired: 10 out]
                n76 = Bundle By Name(cluster=w302, "State Changed?"=w296, "Action Name"=w304) -> (w301:T2)
              }
              frame True {
                n77 = call <vilib>:"Scene Settings.vi"("Control Ref Queue"=w312, "error in (no error)"=w310, "Actual Transform In"=w308, "3D Plot.lvclass in"=w309) -> ("error out"=w316:errorcluster, "Actual Transform Out"=w326:T11, "3D Plot.lvclass out"=w317:refnum<class "3D Comet.lvclass">)  [unwired: 3 in, 2 out]
                n78 = call <vilib>:"Update Scene Object.vi"("Action"=T9 {"Light Action"=enum."Update", "Axis Action"=enum."Update", "Plot Action"=enum."Update", "Cursor Action"=enum."Update", "Fast Draw Action"=enum."Nothing"}, "Control Ref Queue"=w312, "Multiplot Representation In"=w311, "error in (no error)"=w316, "Object Cluster In"=w320, "Actual Transform In"=w326, "3D Plot.lvclass in"=w317) -> ("error out"=w323:errorcluster, "Object Cluster Out"=w327:T16, "Actual Transform Out"=w313:T11, "3D Plot.lvclass out"=w325:refnum<class "3D Comet.lvclass">, "Multiplot Representation Out"=w315:T13)
                n79 = call-dynamic "Graph Color Legend.vi"("Control Ref Queue"=w312, "Multiplot Representation In"=w315, "error in (no error)"=w323, "3D Plot.lvclass in"=w325) -> ("error out"=w319:errorcluster, "3D Plot.lvclass out"=w324:refnum<class "3D Comet.lvclass">, "Multiplot Representation Out"=w314:T13)  [unwired: 2 in, 3 out]
                n80 = invoke on="3D Picture Control" class="SceneGraphDisp (strict)" method="Redraw"(error in=w319) -> (error out=w318:errorcluster)  [unwired: 2 in, 2 out]
                n81 = call <vilib>:"Render Window Redraw.vi"("Control Ref Queue"=w312, "error in (no error)"=w318) -> ()  [unwired: 1 in, 9 out]
              }
            }
            n82 = Bundle By Name(cluster=w295, "3D Comet.lvclass"=w290) -> (w294:T3)
          }
          frame "USER_RENDER_WINDOW" {
            n83 = Unbundle By Name(w331) -> ("Control Ref Queue"=w330:T4)
            n84 = call <vilib>:"Render Window Open.vi"("Control Ref Queue"=w330, "Object Cluster In"=w329) -> ("Object Cluster Out"=w328:T16)  [unwired: 3 in, 6 out]
          }
          frame "USER_EXPORT_IMAGE" {
            n85 = Unbundle By Name(w338) -> ("Control Ref Queue"=w337:T4)
            n86 = call <vilib>:"Image File Dialog.vi"("Control Ref Queue"=w337) -> ()  [unwired: 2 in, 9 out]
          }
          frame "USER_PRINT_IMAGE" {
            n87 = Unbundle By Name(w345) -> ("Control Ref Queue"=w348:T4)
            n88 = call <vilib>:"Image to Printer.vi"("Control Ref Queue"=w348) -> ()  [unwired: 1 in, 10 out]
          }
          frame "USER_PROJECTION_VISIBLE" {
            w362 = T17 1 items=["Attribute", "Show/Hide", "Cursor Move", "Zoom", "Mouse Drag", "XY Projection", "YZ Projection", "XZ Projection", "3D Projection", "Active Plot", "Scale"] ("Global String")
            n89 = Unbundle By Name(w366) -> ("3D Comet.lvclass"=w370:refnum<class "3D Comet.lvclass">, "Control Ref Queue"=w353:T4)
            n90 = call <vilib>:"Read Property.vi"("3D Plot.lvclass in"=w370) -> ("error out"=w355:errorcluster, "Property Cluster"=w368:T18, "3D Plot.lvclass out"=w369:refnum<class "3D Comet.lvclass">)  [unwired: 1 in, 7 out]
            n91 = Unbundle By Name(w368) -> ("Appearance Property.Visibility.Projection Palette"=w372:bool)
            n92 = Not(x=w372) -> (.not. x?=w359:bool)
            n93 = Bundle By Name(cluster=w368, "Appearance Property.Visibility.Projection Palette"=w359) -> (w367:T18)
            n94 = call <vilib>:"3DMathPlot Action String.vi"("Global String"=w362) -> ("String Out"=w361:string)  [unwired: 10 out]
            n95 = call <vilib>:"Write Property.vi"("error in (no error)"=w355, "Property Cluster"=w367, "3D Plot.lvclass in"=w369) -> ("error out"=w358:errorcluster, "3D Plot.lvclass out"=w357:refnum<class "3D Comet.lvclass">)  [unwired: 7 out]
            n96 = Bundle By Name(cluster=w374, "State Changed?"=TRUE ("Data Changed?"), "Action Name"=w361) -> (w373:T2)
            n97 = call <vilib>:"Update Palette with Ramp.vi"("Control Ref Queue"=w353, "error in (no error)"=w358, "3D Plot.lvclass in"=w357) -> ("Ignore the size change?"=w354:bool, "3D Plot.lvclass out"=w356:refnum<class "3D Comet.lvclass">)  [unwired: 7 out]
            n98 = Bundle By Name(cluster=w366, "3D Comet.lvclass"=w356) -> (w365:T3)
          }
          frame "USER_COLOR_RAMP_VISIBLE" {
            w384 = T17 1 items=["Attribute", "Show/Hide", "Cursor Move", "Zoom", "Mouse Drag", "XY Projection", "YZ Projection", "XZ Projection", "3D Projection", "Active Plot", "Scale"] ("Global String")
            n99 = Unbundle By Name(w392) -> ("3D Comet.lvclass"=w396:refnum<class "3D Comet.lvclass">, "Control Ref Queue"=w376:T4)
            n100 = call <vilib>:"Read Property.vi"("3D Plot.lvclass in"=w396) -> ("error out"=w378:errorcluster, "Property Cluster"=w395:T18, "3D Plot.lvclass out"=w382:refnum<class "3D Comet.lvclass">)  [unwired: 1 in, 7 out]
            n101 = Unbundle By Name(w395) -> ("Appearance Property.Visibility.Color Ramp Palette"=w397:bool)
            n102 = Not(x=w397) -> (.not. x?=w385:bool)
            n103 = Bundle By Name(cluster=w395, "Appearance Property.Visibility.Color Ramp Palette"=w385) -> (w394:T18)
            n104 = call <vilib>:"3DMathPlot Action String.vi"("Global String"=w384) -> ("String Out"=w393:string)  [unwired: 10 out]
            n105 = call <vilib>:"Write Property.vi"("error in (no error)"=w378, "Property Cluster"=w394, "3D Plot.lvclass in"=w382) -> ("error out"=w381:errorcluster, "3D Plot.lvclass out"=w380:refnum<class "3D Comet.lvclass">)  [unwired: 7 out]
            n106 = Bundle By Name(cluster=w387, "State Changed?"=TRUE ("Data Changed?"), "Action Name"=w393) -> (w386:T2)
            n107 = call <vilib>:"Update Palette with Ramp.vi"("Control Ref Queue"=w376, "error in (no error)"=w381, "3D Plot.lvclass in"=w380) -> ("Ignore the size change?"=w377:bool, "3D Plot.lvclass out"=w379:refnum<class "3D Comet.lvclass">)  [unwired: 7 out]
            n108 = Bundle By Name(cluster=w392, "3D Comet.lvclass"=w379) -> (w391:T3)
          }
        }
      }
      event "3D Picture Control": Mouse Down {
        n109 = event-data() -> ("PlatMods.Shift"=w414:bool, "Button"=w400:u16, "PlatMods.Ctrl"=w401:bool)  [unwired: 1 out]
        n110 = call <vilib>:"Check Right Click.vi"("Ctrl"=w401, "Button"=w400) -> ("Right Click?"=w399:bool)  [unwired: 9 out]
        n111 = case shown="False" w399 {
          tunnel: w414 -> [_ w452]
          tunnel: w415 -> [w431 w449]
          tunnel: w419 -> [_ w451]
          tunnel: [w431 w432] -> w405
          tunnel: [w430 w447] -> w402
          tunnel: w418 -> [w430 w446]
          tunnel: w413 -> [w429 w445]
          tunnel: [w429 w444] -> w406
          tunnel: w412 -> [w428 w442]
          tunnel: [w428 w442] -> w407
          tunnel: [w427 w443] -> w408
          tunnel: w410 -> [w427 w441]
          tunnel: [w426 w440] -> w409
          tunnel: w411 -> [w426 w439]
          tunnel: w416 -> [w424 w436]
          tunnel: w417 -> [w425 w435]
          tunnel: [w425 w434] -> w403
          tunnel: [w424 w433] -> w404
          frame True {
          }
          frame False {
            n112 = Unbundle By Name(w451) -> ("3D Comet.lvclass"=w450:refnum<class "3D Comet.lvclass">, "Control Ref Queue"=w438:T4)
            n113 = call <vilib>:"Read Property.vi"("3D Plot.lvclass in"=w450) -> ("Property Cluster"=w448:T18, "3D Plot.lvclass out"=w437:refnum<class "3D Comet.lvclass">)  [unwired: 1 in, 8 out]
            n114 = case shown="False" w442 {
              selector: w442 -> [_ w488]
              tunnel: w452 -> [w462 _]
              tunnel: w448 -> [w465 w491]
              tunnel: w449 -> [w470 w484]
              tunnel: [w462 w489] -> w447
              tunnel: w446 -> [_ w489]
              tunnel: w445 -> [w464 _]
              tunnel: [w464 w488] -> w444
              tunnel: [w463 w490] -> w443
              tunnel: w441 -> [w463 _]
              tunnel: [w461 w487] -> w440
              tunnel: w439 -> [_ w487]
              tunnel: w438 -> [w459 _]
              tunnel: w437 -> [w458 _]
              tunnel: w436 -> [w457 w485]
              tunnel: w435 -> [w456 w486]
              tunnel: [w455 w486] -> w434
              tunnel: [w454 w485] -> w433
              tunnel: [w453 w484] -> w432
              frame False {
                n115 = Unbundle By Name(w465) -> ("Graph Property.General Property.Fast Draw?"=w468:bool, "Graph Property.View Property.View Direction"=w469:T10, "Graph Property.View Property.User Defined View Direction.View Distance"=w461:sgl)
                n116 = Equal?(x=w469, y=T10."User Defined") -> (x = y?=w467:bool)
                n117 = And(x=w468, y=w467) -> (x .and. y?=w466:bool)
                n118 = case shown="True" w466 {
                  tunnel: w470 -> [w471 w482]
                  tunnel: w459 -> [_ w481]
                  tunnel: w458 -> [_ w480]
                  tunnel: w457 -> [w472 w479]
                  tunnel: w456 -> [w473 w478]
                  tunnel: [w473 w476] -> w455
                  tunnel: [w472 w475] -> w454
                  tunnel: [w471 w474] -> w453
                  frame False {
                  }
                  frame True {
                    # "Update the Fast Draw and display it."
                    n119 = call <vilib>:"Update Scene Object.vi"("Action"=T9 {"Light Action"=enum."Nothing", "Axis Action"=enum."Nothing", "Plot Action"=enum."Nothing", "Cursor Action"=enum."Nothing", "Fast Draw Action"=enum."Update"}, "Control Ref Queue"=w481, "Multiplot Representation In"=w478, "Object Cluster In"=w482, "Actual Transform In"=w479, "3D Plot.lvclass in"=w480) -> ("Object Cluster Out"=w474:T16, "Actual Transform Out"=w475:T11, "Multiplot Representation Out"=w476:T13)  [unwired: 1 in, 2 out]
                    n120 = Unbundle By Name(w474) -> ("Fast Root Scene Object"=w483:refnum<vi>)
                    n121 = local write "3D Picture Control"(w483) -> ()
                  }
                }
              }
              frame True {
                n122 = Unbundle By Name(w491) -> ("Cursor Property Array"=w490:T34)
              }
            }
          }
        }
      }
      event "3D Picture Control": Mouse Up {
        w498 = FALSE
        n123 = event-data() -> ("Button"=w503:u16)  [unwired: 1 out]
        n124 = case shown="1" w503 {
          tunnel: w506 -> [w514 w549]
          tunnel: w509 -> [w515 w531]
          tunnel: [w513 w539] -> w504
          tunnel: [w515 w536] -> w508
          tunnel: [w514 w548] -> w505
          tunnel: w502 -> [_ w546]
          tunnel: w501 -> [_ w545]
          tunnel: w500 -> [_ w541]
          tunnel: w507 -> [w513 w540]
          tunnel: w497 -> [w512 w525]
          tunnel: [w512 w526] -> w496
          tunnel: w495 -> [w511 w529]
          tunnel: [w511 w527] -> w494
          tunnel: w492 -> [_ w534]
          frame 0, Default {
          }
          frame 1 {
            n125 = Build Array(w546, w545) -> (w544:bool[])
            n126 = Unbundle By Name(w540) -> ("3D Comet.lvclass"=w523:refnum<class "3D Comet.lvclass">, "Control Ref Queue"=w530:T4)
            n127 = Boolean Array To Number(Boolean array=w544) -> (number=w543:u32)
            n128 = call <vilib>:"Read Property.vi"("3D Plot.lvclass in"=w523) -> ("error out"=w517:errorcluster, "Property Cluster"=w520:T18, "3D Plot.lvclass out"=w524:refnum<class "3D Comet.lvclass">)  [unwired: 1 in, 7 out]
            n129 = case shown="2" w543 {
              tunnel: [w557 w563 w568] -> w547
              tunnel: [w552 TRUE ("State Changed?") TRUE ("State Changed?")] -> w542
              tunnel: w541 -> [_ _ w570]
              tunnel: w530 -> [w555 _ _]
              tunnel: w534 -> [_ w561 _]
              tunnel: w520 -> [w554 w560 w567]
              tunnel: [w553 w559 w566] -> w519
              tunnel: w517 -> [w551 w558 w565]
              tunnel: [w550 w558 w565] -> w516
              frame 0, Default {
                w556 = T17 4 items=["Attribute", "Show/Hide", "Cursor Move", "Zoom", "Mouse Drag", "XY Projection", "YZ Projection", "XZ Projection", "3D Projection", "Active Plot", "Scale"] ("Global String")
                n130 = call <vilib>:"Get Latitude & Longitude.vi"("Control Ref Queue"=w555, "error in (no error)"=w551, "Property Cluster in"=w554) -> ("error out"=w550:errorcluster, "State Changed?"=w552:bool, "Property Cluster out"=w553:T18)  [unwired: 6 out]
                n131 = call <vilib>:"3DMathPlot Action String.vi"("Global String"=w556) -> ("String Out"=w557:string)  [unwired: 10 out]
              }
              frame 1 {
                w562 = T17 3 items=["Attribute", "Show/Hide", "Cursor Move", "Zoom", "Mouse Drag", "XY Projection", "YZ Projection", "XZ Projection", "3D Projection", "Active Plot", "Scale"] ("Global String")
                n132 = Bundle By Name(cluster=w560, "Graph Property.View Property.User Defined View Direction.View Distance"=w561) -> (w559:T18)
                n133 = call <vilib>:"3DMathPlot Action String.vi"("Global String"=w562) -> ("String Out"=w563:string)  [unwired: 10 out]
              }
              frame 2 {
                w569 = T17 2 items=["Attribute", "Show/Hide", "Cursor Move", "Zoom", "Mouse Drag", "XY Projection", "YZ Projection", "XZ Projection", "3D Projection", "Active Plot", "Scale"] ("Global String")
                n134 = Bundle By Name(cluster=w567, "Cursor Property Array"=w570) -> (w566:T18)
                n135 = call <vilib>:"3DMathPlot Action String.vi"("Global String"=w569) -> ("String Out"=w568:string)  [unwired: 10 out]
              }
            }
            n136 = call <vilib>:"Write Property.vi"("error in (no error)"=w516, "Property Cluster"=w519, "3D Plot.lvclass in"=w524) -> ("error out"=w521:errorcluster, "3D Plot.lvclass out"=w522:refnum<class "3D Comet.lvclass">)  [unwired: 7 out]
            n137 = call <vilib>:"Scene Settings.vi"("Control Ref Queue"=w530, "error in (no error)"=w521, "Actual Transform In"=w529, "3D Plot.lvclass in"=w522) -> ("error out"=w533:errorcluster, "Actual Transform Out"=w528:T11, "3D Plot.lvclass out"=w532:refnum<class "3D Comet.lvclass">)  [unwired: 3 in, 2 out]
            n138 = call <vilib>:"Update Scene Object.vi"("Action"=T9 {"Light Action"=enum."Nothing", "Axis Action"=enum."Nothing", "Plot Action"=enum."Nothing", "Cursor Action"=enum."Update", "Fast Draw Action"=enum."Nothing"}, "Control Ref Queue"=w530, "Multiplot Representation In"=w525, "error in (no error)"=w533, "Object Cluster In"=w531, "Actual Transform In"=w528, "3D Plot.lvclass in"=w532) -> ("error out"=w535:errorcluster, "Object Cluster Out"=w536:T16, "Actual Transform Out"=w527:T11, "3D Plot.lvclass out"=w518:refnum<class "3D Comet.lvclass">, "Multiplot Representation Out"=w526:T13)
            n139 = Unbundle By Name(w536) -> ("Root Scene Object"=w537:refnum<vi>)
            n140 = call <vilib>:"Render Window Redraw.vi"("Control Ref Queue"=w530, "error in (no error)"=w535) -> ()  [unwired: 1 in, 9 out]
            n141 = Bundle By Name(cluster=w549, "State Changed?"=w542, "Action Name"=w547) -> (w548:T2)
            n142 = local write "3D Picture Control"(w537) -> ()
            n143 = Bundle By Name(cluster=w540, "3D Comet.lvclass"=w518) -> (w539:T3)
          }
        }
      }
      event "3D Picture Control": Mouse Move {
        n144 = event-data() -> ("Coords"=w575:T45)  [unwired: 1 out]
        n145 = Unbundle By Name(w590) -> ("3D Comet.lvclass"=w574:refnum<class "3D Comet.lvclass">, "Control Ref Queue"=w577:T4)
        n146 = call <vilib>:"Plot Zoom.vi"("Control Ref Queue"=w577, "Zoom Mode"=w592, "3D Plot.lvclass in"=w574) -> ("error out"=w589:errorcluster, "Dup Ortho Zoom Mode"=w591:bool, "3D Plot.lvclass out"=w573:refnum<class "3D Comet.lvclass">, "View Distance Out"=w572:sgl)  [unwired: 2 in, 3 out]
        n147 = call <vilib>:"Cursor Move.vi"("3D Plot.lvclass in"=w573, "Coords"=w575, "Control Ref Queue"=w577, "Actual Transform In"=w579, "Object Cluster In"=w588, "Cursor ID In"=w586, "Tracking Cursor?"=w582, "error in (no error)"=w589, "Multiplot Represention"=w580) -> ("Object Cluster Out"=w587:T16, "Cursor ID"=w585:i32, "Drag Cursor?"=w581:bool, "Update Plot?"=w583:bool, "Cursor Property Array"=w584:T34, "error out"=w576:errorcluster)  [unwired: 1 out]
        n148 = case shown="True" w583 {
          tunnel: w576 -> [_ w595]
          frame False {
          }
          frame True {
            n149 = invoke on="3D Picture Control" class="SceneGraphDisp (strict)" method="Redraw"(error in=w595) -> ()  [unwired: 2 in, 3 out]
          }
        }
      }
      event "Projection Palette.XY Projection": Value Change {
        w611 = T17 5 items=["Attribute", "Show/Hide", "Cursor Move", "Zoom", "Mouse Drag", "XY Projection", "YZ Projection", "XZ Projection", "3D Projection", "Active Plot", "Scale"] ("Global String")
        n150 = event-data() -> ("NewVal"=w597:bool)  [unwired: 1 out]
        n151 = Unbundle By Name(w616) -> ("3D Comet.lvclass"=w603:refnum<class "3D Comet.lvclass">, "Control Ref Queue"=w596:T4)
        n152 = call <vilib>:"View Direction Write.vi"("Control Ref Queue"=w596, "View Direction"=T10."Towards X-Y Plane", "3D Plot.lvclass in"=w603) -> ("error out"=w601:errorcluster, "3D Plot.lvclass out"=w602:refnum<class "3D Comet.lvclass">)  [unwired: 1 in, 6 out]
        n153 = call <vilib>:"Scene Settings.vi"("Control Ref Queue"=w596, "error in (no error)"=w601, "Actual Transform In"=w600, "3D Plot.lvclass in"=w602) -> ("error out"=w605:errorcluster, "Actual Transform Out"=w599:T11, "3D Plot.lvclass out"=w607:refnum<class "3D Comet.lvclass">)  [unwired: 3 in, 2 out]
        n154 = call <vilib>:"3DMathPlot Action String.vi"("Global String"=w611) -> ("String Out"=w612:string)  [unwired: 10 out]
        n155 = invoke on="3D Picture Control" class="SceneGraphDisp (strict)" method="Redraw"(error in=w605) -> (error out=w609:errorcluster)  [unwired: 2 in, 2 out]
        n156 = Bundle By Name(cluster=w615, "State Changed?"=w597, "Action Name"=w612) -> (w614:T2)
        n157 = call <vilib>:"Render Window Redraw.vi"("Control Ref Queue"=w596, "error in (no error)"=w609) -> ()  [unwired: 1 in, 9 out]
        n158 = Bundle By Name(cluster=w616, "3D Comet.lvclass"=w607) -> (w613:T3)
      }
      event "Projection Palette.XZ Projection": Value Change {
        w638 = T17 7 items=["Attribute", "Show/Hide", "Cursor Move", "Zoom", "Mouse Drag", "XY Projection", "YZ Projection", "XZ Projection", "3D Projection", "Active Plot", "Scale"] ("Global String")
        n159 = event-data() -> ("NewVal"=w624:bool)  [unwired: 1 out]
        n160 = Unbundle By Name(w643) -> ("3D Comet.lvclass"=w628:refnum<class "3D Comet.lvclass">, "Control Ref Queue"=w623:T4)
        n161 = call <vilib>:"View Direction Write.vi"("Control Ref Queue"=w623, "View Direction"=T10."Towards X-Z Plane", "3D Plot.lvclass in"=w628) -> ("error out"=w626:errorcluster, "3D Plot.lvclass out"=w627:refnum<class "3D Comet.lvclass">)  [unwired: 1 in, 6 out]
        n162 = call <vilib>:"Scene Settings.vi"("Control Ref Queue"=w623, "error in (no error)"=w626, "Actual Transform In"=w630, "3D Plot.lvclass in"=w627) -> ("error out"=w632:errorcluster, "Actual Transform Out"=w629:T11, "3D Plot.lvclass out"=w633:refnum<class "3D Comet.lvclass">)  [unwired: 4 in, 1 out]
        n163 = call <vilib>:"3DMathPlot Action String.vi"("Global String"=w638) -> ("String Out"=w639:string)  [unwired: 10 out]
        n164 = invoke on="3D Picture Control" class="SceneGraphDisp (strict)" method="Redraw"(error in=w632) -> (error out=w636:errorcluster)  [unwired: 2 in, 2 out]
        n165 = Bundle By Name(cluster=w641, "State Changed?"=w624, "Action Name"=w639) -> (w640:T2)
        n166 = call <vilib>:"Render Window Redraw.vi"("Control Ref Queue"=w623, "error in (no error)"=w636) -> ()  [unwired: 1 in, 9 out]
        n167 = Bundle By Name(cluster=w643, "3D Comet.lvclass"=w633) -> (w642:T3)
      }
      event "Projection Palette.YZ Projection": Value Change {
        w665 = T17 6 items=["Attribute", "Show/Hide", "Cursor Move", "Zoom", "Mouse Drag", "XY Projection", "YZ Projection", "XZ Projection", "3D Projection", "Active Plot", "Scale"] ("Global String")
        n168 = event-data() -> ("NewVal"=w651:bool)  [unwired: 1 out]
        n169 = Unbundle By Name(w670) -> ("3D Comet.lvclass"=w655:refnum<class "3D Comet.lvclass">, "Control Ref Queue"=w650:T4)
        n170 = call <vilib>:"View Direction Write.vi"("Control Ref Queue"=w650, "View Direction"=T10."Towards Y-Z Plane", "3D Plot.lvclass in"=w655) -> ("error out"=w653:errorcluster, "3D Plot.lvclass out"=w654:refnum<class "3D Comet.lvclass">)  [unwired: 1 in, 6 out]
        n171 = call <vilib>:"Scene Settings.vi"("Control Ref Queue"=w650, "error in (no error)"=w653, "Actual Transform In"=w657, "3D Plot.lvclass in"=w654) -> ("error out"=w659:errorcluster, "Actual Transform Out"=w656:T11, "3D Plot.lvclass out"=w661:refnum<class "3D Comet.lvclass">)  [unwired: 3 in, 2 out]
        n172 = call <vilib>:"3DMathPlot Action String.vi"("Global String"=w665) -> ("String Out"=w666:string)  [unwired: 10 out]
        n173 = invoke on="3D Picture Control" class="SceneGraphDisp (strict)" method="Redraw"(error in=w659) -> (error out=w663:errorcluster)  [unwired: 2 in, 2 out]
        n174 = Bundle By Name(cluster=w668, "State Changed?"=w651, "Action Name"=w666) -> (w667:T2)
        n175 = call <vilib>:"Render Window Redraw.vi"("Control Ref Queue"=w650, "error in (no error)"=w663) -> ()  [unwired: 1 in, 9 out]
        n176 = Bundle By Name(cluster=w670, "3D Comet.lvclass"=w661) -> (w669:T3)
      }
      event "Projection Palette.3D Projection": Value Change {
        w692 = T17 8 items=["Attribute", "Show/Hide", "Cursor Move", "Zoom", "Mouse Drag", "XY Projection", "YZ Projection", "XZ Projection", "3D Projection", "Active Plot", "Scale"] ("Global String")
        n177 = event-data() -> ("NewVal"=w678:bool)  [unwired: 1 out]
        n178 = Unbundle By Name(w697) -> ("3D Comet.lvclass"=w682:refnum<class "3D Comet.lvclass">, "Control Ref Queue"=w677:T4)
        n179 = call <vilib>:"View Direction Write.vi"("Control Ref Queue"=w677, "View Direction"=T10."User Defined", "3D Plot.lvclass in"=w682) -> ("error out"=w680:errorcluster, "3D Plot.lvclass out"=w681:refnum<class "3D Comet.lvclass">)  [unwired: 1 in, 6 out]
        n180 = call <vilib>:"Scene Settings.vi"("Control Ref Queue"=w677, "error in (no error)"=w680, "Actual Transform In"=w684, "3D Plot.lvclass in"=w681) -> ("error out"=w687:errorcluster, "Actual Transform Out"=w683:T11, "3D Plot.lvclass out"=w686:refnum<class "3D Comet.lvclass">)  [unwired: 3 in, 2 out]
        n181 = call <vilib>:"3DMathPlot Action String.vi"("Global String"=w692) -> ("String Out"=w693:string)  [unwired: 10 out]
        n182 = invoke on="3D Picture Control" class="SceneGraphDisp (strict)" method="Redraw"(error in=w687) -> (error out=w690:errorcluster)  [unwired: 2 in, 2 out]
        n183 = Bundle By Name(cluster=w695, "State Changed?"=w678, "Action Name"=w693) -> (w694:T2)
        n184 = call <vilib>:"Render Window Redraw.vi"("Control Ref Queue"=w677, "error in (no error)"=w690) -> ()  [unwired: 1 in, 9 out]
        n185 = Bundle By Name(cluster=w697, "3D Comet.lvclass"=w686) -> (w696:T3)
      }
      event "Color Ramp Palette.Active Plot": Value Change {
        w716 = T17 9 items=["Attribute", "Show/Hide", "Cursor Move", "Zoom", "Mouse Drag", "XY Projection", "YZ Projection", "XZ Projection", "3D Projection", "Active Plot", "Scale"] ("Global String")
        n186 = event-data() -> ("NewVal"=w719:i32)  [unwired: 1 out]
        n187 = Unbundle By Name(w721) -> ("3D Comet.lvclass"=w722:refnum<class "3D Comet.lvclass">, "Control Ref Queue"=w711:T4)
        n188 = call-dynamic "Write Active Plot.vi"("Active Plot"=w719, "3D Comet.lvclass in"=w722) -> ("error out"=w706:errorcluster, "3D Comet.lvclass out"=w707:refnum<class "3D Comet.lvclass">)  [unwired: 8 in]
        n189 = call <vilib>:"3DMathPlot Action String.vi"("Global String"=w716) -> ("String Out"=w717:string)  [unwired: 10 out]
        n190 = Bundle By Name(cluster=w715, "State Changed?"=TRUE ("Data Changed?"), "Action Name"=w717) -> (w714:T2)
        n191 = call-dynamic "Graph Color Legend.vi"("Control Ref Queue"=w711, "Multiplot Representation In"=w705, "error in (no error)"=w706, "3D Plot.lvclass in"=w707) -> ("3D Plot.lvclass out"=w713:refnum<class "3D Comet.lvclass">, "Multiplot Representation Out"=w704:T13)  [unwired: 2 in, 4 out]
        n192 = Bundle By Name(cluster=w721, "3D Comet.lvclass"=w713) -> (w720:T3)
      }
      event "XY Graph": Scale Range Change {
        w744 = T17 10 items=["Attribute", "Show/Hide", "Cursor Move", "Zoom", "Mouse Drag", "XY Projection", "YZ Projection", "XZ Projection", "3D Projection", "Active Plot", "Scale"] ("Global String")
        n193 = event-data() -> ("NewRange"=w755:T46, "Kind"=w754:enum16{"X-Scale", "Y-Scale", "Z-Scale"})  [unwired: 1 out]
        n194 = Unbundle By Name(w752) -> ("3D Comet.lvclass"=w753:refnum<class "3D Comet.lvclass">, "Control Ref Queue"=w737:T4)
        n195 = call <vilib>:"Transform Cluster Update.vi"("Axis"=w754, "NewRange"=w755, "Multiplot Representation In"=w730, "Actual Transform In"=w733, "3D Plot in"=w753) -> ("error out"=w739:errorcluster, "Actual Transform Out"=w732:T11, "3D Plot out"=w740:refnum<class "3D Comet.lvclass">, "Multiplot Representation Out"=w731:T13)  [unwired: 1 in, 2 out]
        n196 = call <vilib>:"Update Scene Object.vi"("Action"=T9 {"Light Action"=enum."Nothing", "Axis Action"=enum."Update", "Plot Action"=enum."Update", "Cursor Action"=enum."Update", "Fast Draw Action"=enum."Nothing"}, "Control Ref Queue"=w737, "Multiplot Representation In"=w731, "error in (no error)"=w739, "Object Cluster In"=w746, "Actual Transform In"=w732, "3D Plot.lvclass in"=w740) -> ("error out"=w741:errorcluster, "Object Cluster Out"=w747:T16, "Actual Transform Out"=w735:T11, "3D Plot.lvclass out"=w729:refnum<class "3D Comet.lvclass">, "Multiplot Representation Out"=w734:T13)
        n197 = invoke on="3D Picture Control" class="SceneGraphDisp (strict)" method="Redraw"(error in=w741) -> (error out=w738:errorcluster)  [unwired: 2 in, 2 out]
        n198 = call <vilib>:"3DMathPlot Action String.vi"("Global String"=w744) -> ("String Out"=w745:string)  [unwired: 10 out]
        n199 = call <vilib>:"Render Window Redraw.vi"("Control Ref Queue"=w737, "error in (no error)"=w738) -> ()  [unwired: 1 in, 9 out]
        n200 = Bundle By Name(cluster=w749, "State Changed?"=TRUE ("Data Changed?"), "Action Name"=w745) -> (w748:T2)
        n201 = Bundle By Name(cluster=w752, "3D Comet.lvclass"=w729) -> (w751:T3)
      }
      event Panel Resize {
        n202 = event-data() -> ()  [unwired: 2 out]
        n203 = case shown="False" w766 {
          tunnel: w768 -> [w781 w783]
          tunnel: [w780 w783] -> w767
          frame False {
            n204 = Unbundle By Name(w781) -> ("3D Comet.lvclass"=w782:refnum<class "3D Comet.lvclass">, "Control Ref Queue"=w779:T4)
            n205 = call <vilib>:"Panel Resize.vi"("Control Ref Queue"=w779, "3D Plot.lvclass"=w782) -> ("error out"=w777:errorcluster, "3D Plot.lvclass out"=w778:refnum<class "3D Comet.lvclass">)  [unwired: 3 in, 5 out]
            n206 = invoke on="3D Picture Control" class="SceneGraphDisp (strict)" method="Redraw"(error in=w777) -> ()  [unwired: 2 in, 3 out]
            n207 = Bundle By Name(cluster=w781, "3D Comet.lvclass"=w778) -> (w780:T3)
          }
          frame True {
          }
        }
      }
    }
  }
  "Display State Out" <- w7
  "Data Out" <- w9
  "Action" <- w6
